vi "FL24 Dryer Tool Main.vi"() -> ()   [LabVIEW 2016]
uses:
  Q:/Common/LabVIEW GEA2 Toolkit/LabVIEW_GEA2_Toolkit.lvlibp/type defs/Data In.ctl
  Q:/Common/LabVIEW GEA2 Toolkit/LabVIEW_GEA2_Toolkit.lvlibp/type defs/Source_Destination.ctl
  Q:/Common/LabVIEW GEA2 Toolkit/LabVIEW_GEA2_Toolkit.lvlibp/type defs/Data Type.ctl
  Q:/Common/LabVIEW GEA2 Toolkit/LabVIEW_GEA2_Toolkit.lvlibp/type defs/ERD Read Data In.ctl
  Q:/MyWork/TL24 Tool/Laundry Tool 2.0 Support/type defs2/Select _Graph_Brass.ctl
  Q:/MyWork/TL24 Tool/Laundry Tool 1.0 Support/type defs/ERD_Graph_All.ctl
  Q:/MyWork/TL24 Tool/Laundry Tool 1.0 Support/type defs/ERD_Graph.ctl
  Q:/MyWork/TL24 Tool/Laundry Tool 1.0 Support/type defs/Version.ctl
  Q:/MyWork/TL24 Tool/Laundry Tool 2.0 Support/type defs2/ERD_Always_Show_Brass.ctl
  Q:/MyWork/TL24 Tool/Laundry Tool 1.0 Support/type defs/Fault_Buffer_Status.ctl
  Q:/MyWork/TL24 Tool/Laundry Tool 2.0 Support/type defs2/Diagnostics_Table.ctl
  Q:/MyWork/TL24 Tool/Laundry Tool 1.0 Support/type defs/Cycle_Diag_Buffer_Status.ctl
  Q:/MyWork/TL24 Tool/Laundry Tool 2.0 Support/type defs2/ERD_Data_Loop_Control_Brass.ctl
  Q:/MyWork/TL24 Tool/Laundry Tool 2.0 Support/type defs2/ERD_Loop_States_Brass.ctl
  Q:/MyWork/TL24 Tool/Laundry Tool 2.0 Support/type defs2/Error_Command_Brass.ctl
  Q:/MyWork/TL24 Tool/Laundry Tool 2.0 Support/type defs2/DAQ_States_Brass.ctl
  Q:/Common/GExplorer Support/typedefs/GExplorer_Data_Cluster.ctl
  Q:/MyWork/TL24 Tool/Laundry Tool 1.0 Support/type defs/Cont_Send_States.ctl
  Q:/MyWork/TL24 Tool/Laundry Tool 2.0 Support/type defs2/Cont_Send_States_Brass.ctl
  Q:/Common/LabVIEW GEA2 Toolkit/LabVIEW_GEA2_Toolkit.lvlibp/type defs/Data Out.ctl
  Q:/Common/LabVIEW GEA2 Toolkit/LabVIEW_GEA2_Toolkit.lvlibp/type defs/ERD Write Data In.ctl
  Q:/MyWork/TL24 Tool/Laundry Tool 2.0 Support/type defs2/DAQ_Control_Command_Brass.ctl
  Q:/MyWork/TL24 Tool/Laundry Tool 2.0 Support/type defs2/ERD_Loop_Control_Command_Brass.ctl
  Q:/MyWork/TL24 Tool/Laundry Tool 2.0 Support/type defs2/GEA2_Control_Command_Brass.ctl
  <vilib>/DAQmx/read.llb/DAQmx Read (Digital 1D Bool NChan 1Samp 1Line).vi
  <vilib>/DAQmx/read.llb/DAQmx Read (Digital 1D U8 1Chan NSamp).vi
  <vilib>/DAQmx/write.llb/DAQmx Write (Digital Bool 1Line 1Point).vi
  <vilib>/DAQmx/read.llb/DAQmx Read (Counter U32 1Chan 1Samp).vi
  <vilib>/DAQmx/write.llb/DAQmx Write (Analog 1D DBL NChan 1Samp).vi
  <vilib>/DAQmx/write.llb/DAQmx Write (Digital 1D Bool NChan 1Samp 1Line).vi
  Q:/Common/LabVIEW GEA2 Toolkit/LabVIEW_GEA2_Toolkit.lvlibp/advanced/GEA2 Message Received Event Handler.vi
  <vilib>/DAQmx/create/channels.llb/DAQmx Create Channel (DO-Digital Output).vi
  <vilib>/DAQmx/create/channels.llb/DAQmx Create Channel (DI-Digital Input).vi
  <vilib>/DAQmx/configure/timing.llb/DAQmx Timing (Sample Clock).vi
  <vilib>/DAQmx/create/channels.llb/DAQmx Create Channel (CO-Pulse Generation-Frequency).vi
  <vilib>/DAQmx/configure/timing.llb/DAQmx Timing (Implicit).vi
  <vilib>/DAQmx/create/channels.llb/DAQmx Create Channel (CI-Count Edges).vi
  <vilib>/DAQmx/create/channels.llb/DAQmx Create Channel (AO-Voltage-Basic).vi
  <vilib>/DAQmx/miscellaneous.llb/DAQmx Fill In Error Info.vi
  C:/Automation/DLLs/PC Dot Net/GeaCommunication.dll
  Automation/DLLs/PC Dot Net/GeaCommunication.dll
  Q:/Common/LabVIEW GEA2 Toolkit/LabVIEW_GEA2_Toolkit.lvlibp
  Q:/Automation/Product Specific/Clothes Care/2015 VA Washer/Projects/2015 VA Washer.lvlib
  <resource>/objmgr/daqmx.rc
panel:
  in  "Data ON":bool=TRUE
  out "ERD_Always Show":T1
  in  "Stop":bool
  out "Fault Status":bool
  out "Log Rate (ms)":u32
  in  "Tab Control":T2(tab)
  in  "Filter Data":bool=TRUE
  in  "Start Send":bool
  in  "Cmd":string
  in  "Filter Log":bool
  in  "Msg Rate (ms)":u32=1000 min=50 step=50
  out "CSV File Log Path":path=path "C:/Users/502129737/Desktop/1"
  in  "Clear":bool
  out "GEA2 Log":string
  in  "Board Index":u8 max=0 step=1
  out "Board ID":string="0"
  in  "GEA2 Send":T3={"Source"=228, "Destination"=53, "Command"=0, "Message"=""} {"Command" format="%02x"; "Destination" format="%02x"; "Source" format="%02x"}
  in  "Send Button":bool
  in  "GEA2 Log Length":i32=100000
  in  "Save Log":bool
  out "Version":T4
  in  "GEA Inputs":T5={"Source"=228, "Destination"=53} {"Destination" format="%.0x"; "Source" format="%.0x"}
  in  "Read ERD List":T6[](array[typedef])=[{"ERD Number"=0, "Data Type"=enum."string"}] {"ERD Number" format="%.0x"}
  out "Read ERD Data Out":cluster{"ERD Number":u16, "Data":string}[](array[cluster]) {"ERD Number" format="%.0x"}
  in  "Read ERD":bool
  in  "Write ERD":bool
  in  "Write ERD List":T8(array[cluster])=[{"ERD Number"=0, "Data Type"=enum."string", "Data"=""}] {"ERD Number" format="%.0x"}
  out "All Loads":u16[][](graph)=[[0, 100, 200, 300, 400]]
  in  "ERD Graphing ON":bool
  out "ERD Graph  Ind":T9
  in  "ERD Graph Cntrl":T10={"ERD 3"={"ERD #"=62250, "Data Type"=enum."uint16_t", "Scaler"=32}, "ERD 2"={"ERD #"=62250, "Data Type"=enum."uint16_t", "Scaler"=32}, "ERD 1"={"ERD #"=62250, "Data Type"=enum."uint16_t", "Scaler"=32}} {"ERD 1"."Scaler" min=1; "ERD 1"."ERD #" format="%.0x"; "ERD 2"."Scaler" min=1; "ERD 2"."ERD #" format="%.0x"; "ERD 3"."Scaler" min=1; "ERD 3"."ERD #" format="%.0x"}
  in  "Graphing ON":bool=TRUE
  in  "Select Graph":T12
  out "ERD 3":dbl(graph)
  out "ERD 2":dbl(graph)
  out "ERD 1":dbl(graph)
  in  "Save Fault Log":bool
  in  "Clear Fault Table Buffer":bool
  in  "Clear Fault Seq Buffer":bool
  in  "Fault ON":bool
  out "Fault Table Buffer":string[][](table)
  out "Fault Sequence Buffer":string
  out "Seq Buffer Status":T13
  out "Table Buffer Status":T13
  in  "Save Cycle History Log":bool
  in  "Clear Cycle Buffer":bool
  out "Cycle Buffer Status":T14
  in  "Get Cycle History":bool
  out "Diagnostics Table":T15
  in  "Test Mode":cluster{"Exit":bool, "Enter":bool}
  in  "Lid Lock":cluster{"Lock Lid":bool, "Unlock Lid":bool}
  in  "HE/LE ?":enum16{"HE", "LE"}(ring)
  in  "LL (M - A)":bool=TRUE
  in  "Lid Lock Feedback":bool
  in  "MS (M - A)":bool=TRUE
  out "DAQ Status":string
  out "Drain Pump":bool
  out "Mode Shift":bool
  out "Recirc Pump":bool
  out "Cold Valve":bool
  out "Hot Valve":bool
  out "Spray/Rinse Valve":bool
  out "Fabric SoftValve":bool
  in  "AC Power":bool=TRUE
  in  "Mode Shift FB":bool
  in  "Lid Status":bool=TRUE
  in  "Pressure":dbl(slide) min=0.0 max=5.0 step=0.5 scale=0.0..5.0 scale format="%#_3g"
  in  "Motor Current":dbl(slide)=2.5 min=0.0 max=5.0 step=0.5 scale=0.0..5.0 scale format="%#_3g"
  in  "Turn On DAQ":bool
  out "DAQ On?":bool
  in  "Basket RPM":dbl=1.0 min=1.0 max=800.0 step=5.0
  in  "Temperature":dbl(slide)=2.5 min=0.0 max=5.0 step=0.5 scale=0.0..5.0 scale format="%#_3g"
  out "Triac CW":bool
  out "Traic CCW":bool
  out "CCW":u32
  out "CW":u32
  in  "ERD Read List":T16(array[cluster])=[{"Boolean"=TRUE, "ERD Number"=1, "ERD Name"="Model Number", "Data Type"=enum."string"}, {"Boolean"=TRUE, "ERD Number"=2, "ERD Name"="Serial Number", "Data Type"=enum."string"}, {"Boolean"=TRUE, "ERD Number"=8192, "ERD Name"="Machine Status", "Data Type"=enum."uint8_t"}, {"Boolean"=TRUE, "ERD Number"=8202, "ERD Name"="Cycle Name", "Data Type"=enum."string"}, {"Boolean"=TRUE, "ERD Number"=142, "ERD Name"="Cycle Count", "Data Type"=enum."uint32_t"}, {"Boolean"=TRUE, "ERD Number"=8193, "ERD Name"="Sub-Cycle", "Data Type"=enum."string"}, {"Boolean"=TRUE, "ERD Number"=141, "ERD Name"="System Runtime", "Data Type"=enum."uint32_t"}, {"Boolean"=TRUE, "ERD Number"=8208, "ERD Name"="Delay Time", "Data Type"=enum."uint16_t"}, {"Boolean"=FALSE, "ERD Number"=256, "ERD Name"="Version", "Data Type"=enum."string"}, {"Boolean"=TRUE, "ERD Number"=70, "ERD Name"="Cycle Time", "Data Type"=enum."uint16_t"}, {"Boolean"=TRUE, "ERD Number"=8206, "ERD Name"="Operating Mode", "Data Type"=enum."string"}, {"Boolean"=TRUE, "ERD Number"=8210, "ERD Name"="Door Status", "Data Type"=enum."string"}, {"Boolean"=TRUE, "ERD Number"=8217, "ERD Name"="Temp Level", "Data Type"=enum."string"}, {"Boolean"=TRUE, "ERD Number"=8218, "ERD Name"="Dryness Level", "Data Type"=enum."string"}, {"Boolean"=TRUE, "ERD Number"=8219, "ERD Name"="Extended Tumble", "Data Type"=enum."string"}, {"Boolean"=TRUE, "ERD Number"=61445, "ERD Name"="Input Status", "Data Type"=enum."string"}, {"Boolean"=TRUE, "ERD Number"=61444, "ERD Name"="Dryer Type", "Data Type"=enum."string"}] {"ERD Number" format="%.0x"}
  out "Error Out":errorcluster
  in  "Error In":errorcluster
  # "Software Version"
  # "UI"
  # "MC"
  # "Must input a valid ERD# and Data Type\nDO NOT Leave Blank \nIf no scaler use value of 01"
  # "Contact:\n\nDerek Hibdon\nderek.hibdon@ge.com"
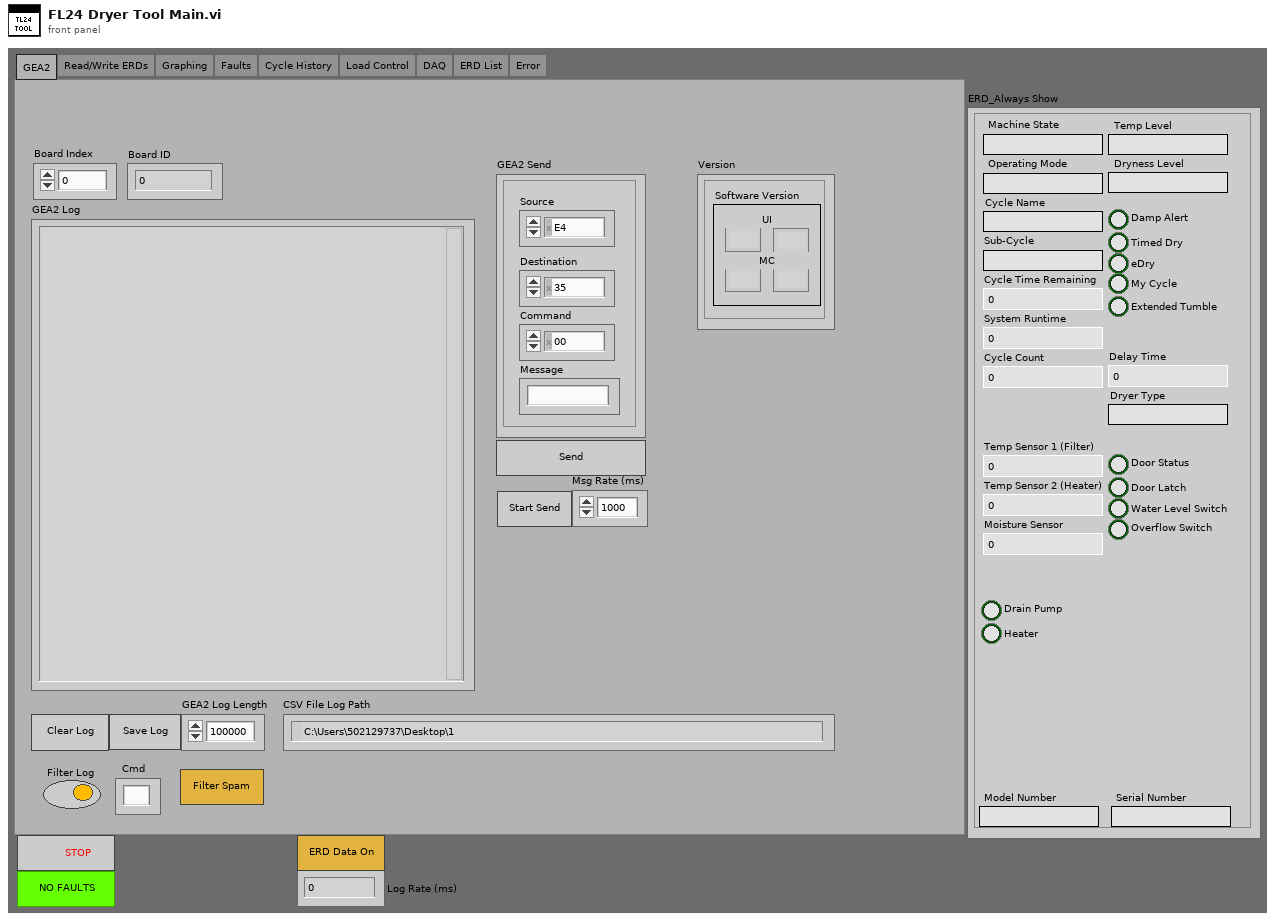
[diagram p1: front panel]
types:
  T1 = typedef "ERD_Always_Show_Brass.ctl" = cluster{"Machine State":string, "Cycle Count":u32, "Dryness Level":string, "Temp Level":string, "Delay Time":u16, "Sub-Cycle":string, "Cycle Name":string, "Model Number":string, "Serial Number":string, "System Runtime":u32, "Cycle Time Remaining":u16, "Operating Mode":string, "Temp Sensor 1 (Filter)":u16, "Drain Pump":bool, "Water Level Switch":bool, "Overflow Switch":bool, "Door Status":bool, "Door Latch":bool, "Heater":bool, "Temp Sensor 2 (Heater)":u16, "Moisture Sensor":u16, "Dryer Type":string, "eDry":bool, "Damp Alert":bool, "Timed Dry":bool, "My Cycle":bool, "Extended Tumble":bool}
  T2 = enum32{"GEA2", "Read/Write ERDs", "Graphing", "Faults", "Cycle History", "Load Control", "DAQ", "ERD List", "Error"}
  T3 = typedef "LabVIEW_GEA2_Toolkit.lvlibp/Data In.ctl" = cluster{"Source":u8, "Destination":u8, "Command":u8, "Message":string}
  T4 = typedef "Version.ctl" = cluster{"Critical Major":string, "Critical Minor":string, "Non-Critical Minor":string, "Non-Critical Major":string}
  T5 = typedef "LabVIEW_GEA2_Toolkit.lvlibp/Source_Destination.ctl" = cluster{"Source":u8, "Destination":u8}
  T6 = typedef "LabVIEW_GEA2_Toolkit.lvlibp/ERD Read Data In.ctl" = cluster{"ERD Number":u16, "Data Type":T7}
  T7 = typedef "LabVIEW_GEA2_Toolkit.lvlibp/Data Type.ctl" = enum16{"string", "boolean", "uint8_t", "uint16_t", "uint32_t", "uint64_t", "int8_t", "int16_t", "int32_t", "int64_t"}
  T8 = cluster{"ERD Number":u16, "Data Type":T7, "Data":string}[]
  T9 = cluster{"ERD Value 1":dbl, "ERD Value 2":dbl, "ERD Value 3":dbl}
  T10 = typedef "ERD_Graph_All.ctl" = cluster{"ERD 3":T11, "ERD 2":T11, "ERD 1":T11}
  T11 = typedef "ERD_Graph.ctl" = cluster{"ERD #":u16, "Data Type":T7, "Scaler":u32}
  T12 = typedef "Select _Graph_Brass.ctl" = enum16{"All Loads", "ERD 1", "ERD 2", "ERD 3", "Temperature (F)", "Basket Speed (RPM)", "Tub Volume (Gal)", "Pressure (in H2O)", "Current RMS (Amps)"}
  T13 = typedef "Fault_Buffer_Status.ctl" = cluster{"Current Index":u16, "Count":u16, "Overwrite Count":u16}
  T14 = typedef "Cycle_Diag_Buffer_Status.ctl" = cluster{"Current Index":u16, "Count":u16, "Overwrite Count":u16}
  T15 = typedef "Diagnostics_Table.ctl" = string[][]
  T16 = cluster{"Boolean":bool, "ERD Number":u16, "ERD Name":string, "Data Type":enum16{"string", "boolean", "uint8_t", "uint16_t", "uint32_t", "uint64_t"}}[]
  T17 = typedef "Cont_Send_States_Brass.ctl" = enum16{"Run", "Shutdown"}
  T18 = typedef "Cont_Send_States.ctl" = enum16{"Run", "Shutdown"}
  T19 = typedef "GExplorer_Data_Cluster.ctl" = cluster{"Data":variant, "State":enum16{"Add to Log", "Clear", "Shutdown"}}
  T20 = typedef "DAQ_States_Brass.ctl" = enum16{"Wait for Init", "Rename Devices", "Verify Hardware", "Initialize", "Run", "Shutdown", "Exit"}
  T21 = typedef "ERD_Data_Loop_Control_Brass.ctl" = cluster{"Data":variant, "State":T22}
  T22 = typedef "ERD_Loop_States_Brass.ctl" = enum16{"Init", "Build ERD Read List", "Read ERDs", "Update UI", "Update Graphs", "Read Faults", "Log Data", "Pause", "Shutdown"}
  T23 = typedef "Error_Command_Brass.ctl" = enum16{"Initialize", "Handle Errors", "Report Errors"}
  T24 = typedef "LabVIEW_GEA2_Toolkit.lvlibp/ERD Write Data In.ctl" = cluster{"ERD Number":u16, "Data Type":T7, "Data":string}
  T25 = typedef "GEA2_Control_Command_Brass.ctl" = enum16{"Initialize", "Shutdown"}
  T26 = typedef "ERD_Loop_Control_Command_Brass.ctl" = enum16{"Initialize", "Shutdown"}
  T27 = typedef "DAQ_Control_Command_Brass.ctl" = enum16{"Initialize", "Shutdown", "Exit"}
  T28 = enum8{"Enabled", "Disabled", "Disabled and Grayed Out"}
  T29 = typedef "LabVIEW_GEA2_Toolkit.lvlibp/Data Out.ctl" = cluster{"Source":u8, "Destination":u8, "Command":u8, "Length":u8, "CRC":u16, "Message":string}
  T30 = typedef "LabVIEW_GEA2_Toolkit.lvlibp/ERD Read Data Out.ctl" = cluster{"ERD Number":u16, "Data":string}
  T31 = typedef "All_Bundled_Data_Brass.ctl" = cluster{"Version":T4, "ERD_Always Show":T1, "Personality Set":u8, "CSV File String Arrays":T32, "Fault Table Array ":T33}
  T32 = typedef "CSV_File_String_Arrays.ctl" = cluster{"ERD Number Array":string[], "ERD Name Array":string[], "ERD Converted String Data":string[]}
  T33 = typedef "Fault Table Array.ctl" = T34[]
  T34 = typedef "Fault_Table_Info.ctl" = cluster{"Cycle Count":u32, " Runtime (min) ":u32, "Fault Status":string, "Fault ID":string, "Fault Count":u16}
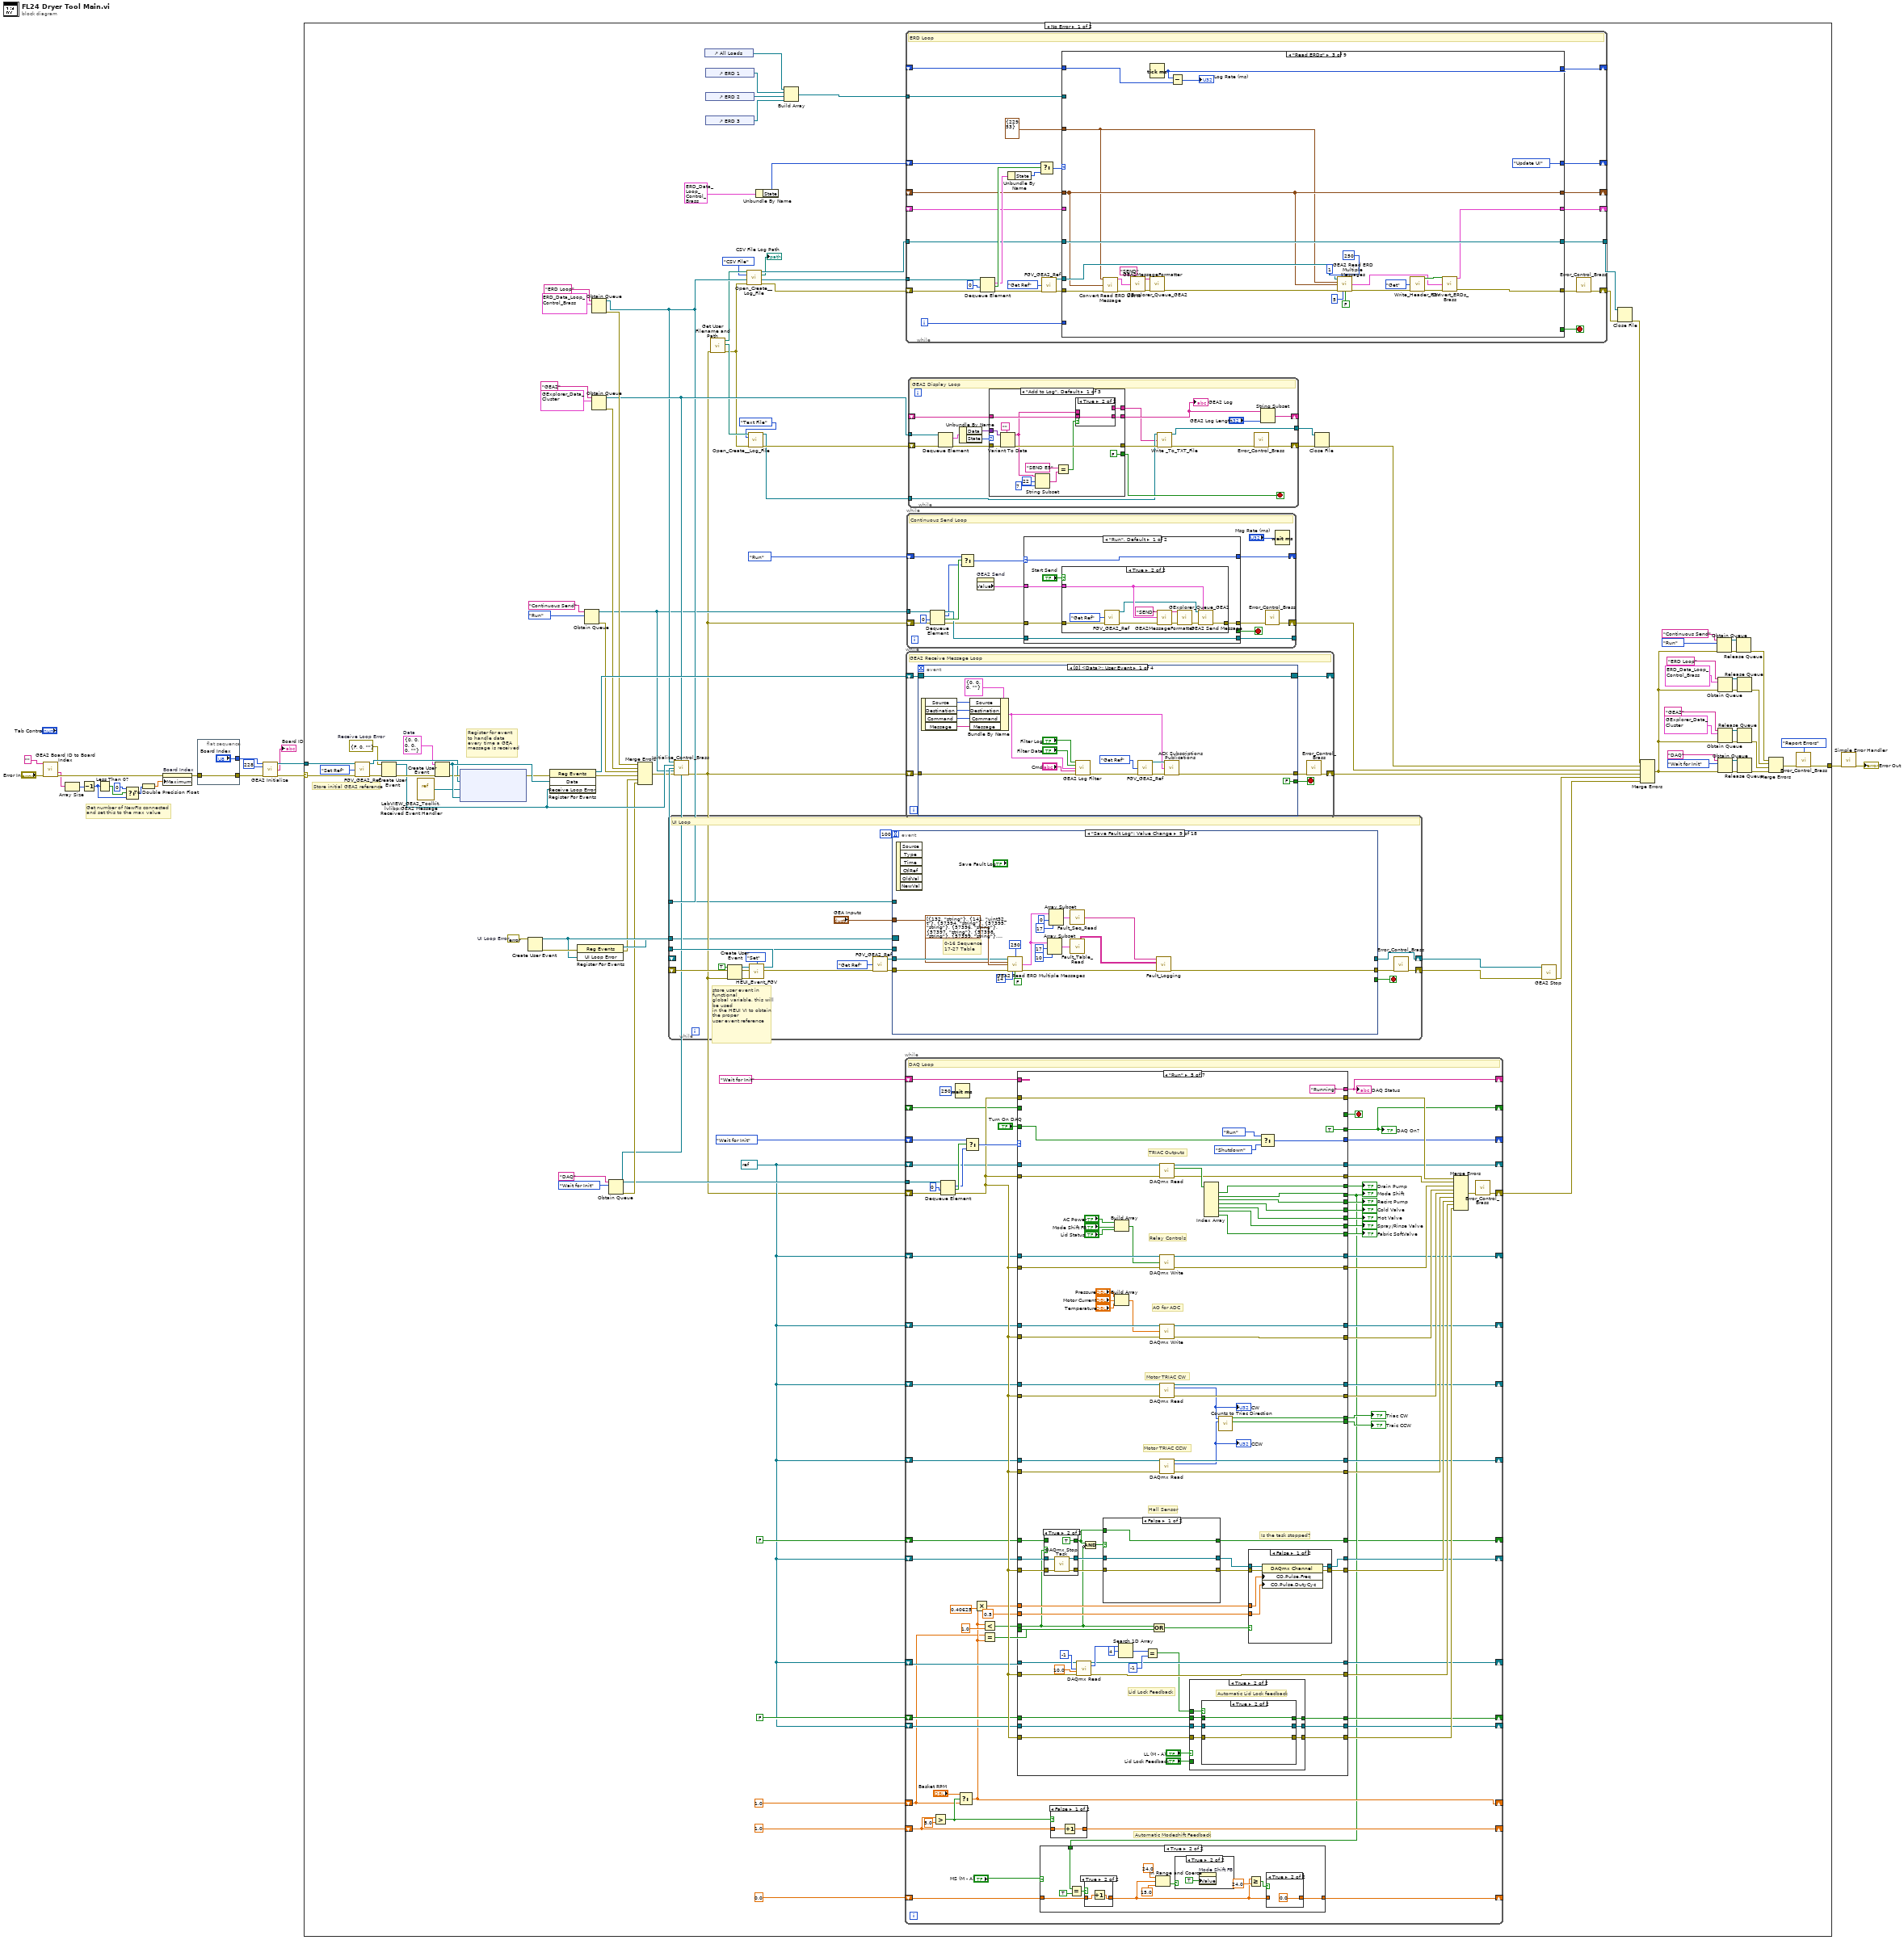
[diagram p0: block diagram]
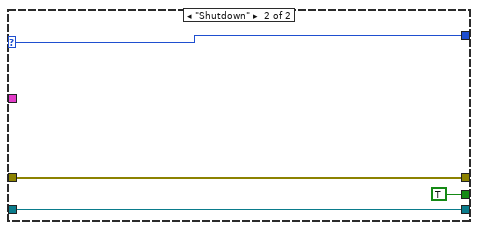
[diagram p3: hidden frame]
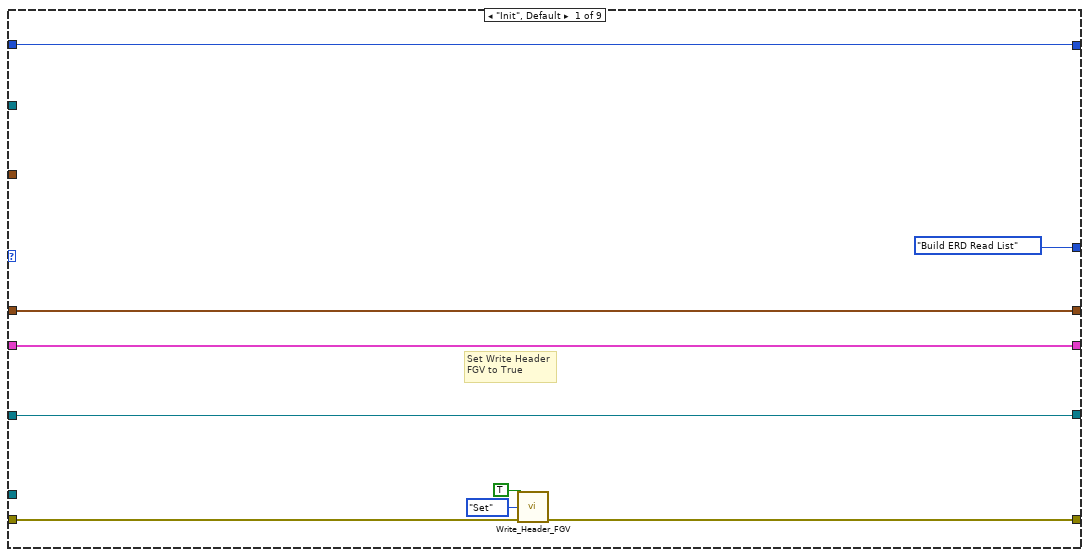
[diagram p4: hidden frame]
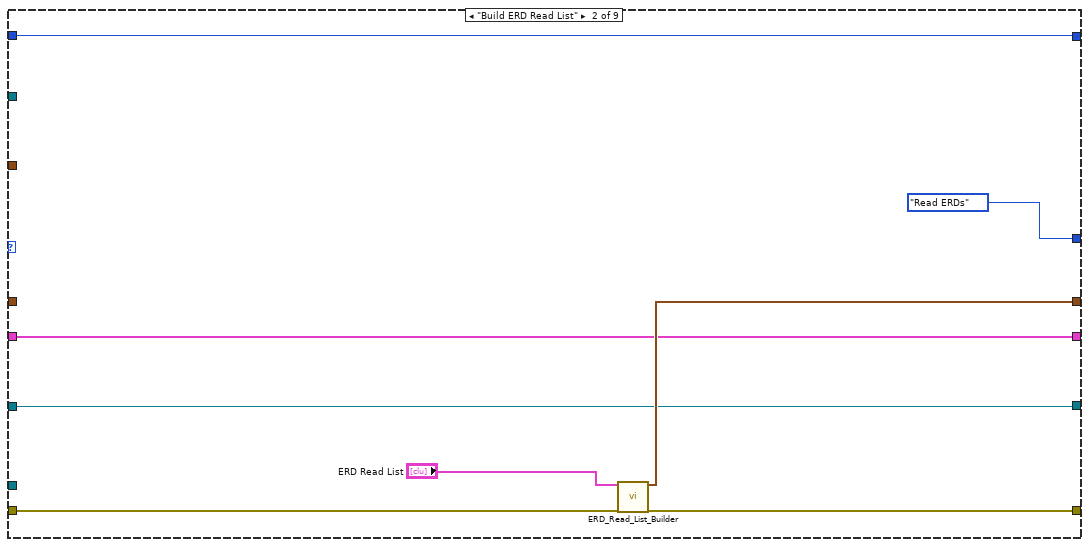
[diagram p5: hidden frame]
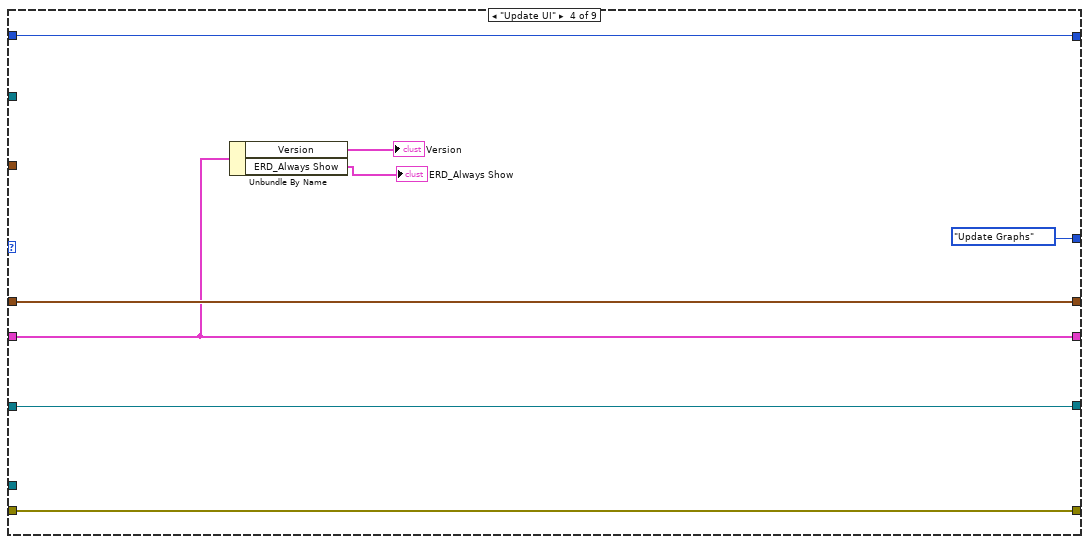
[diagram p6: hidden frame]
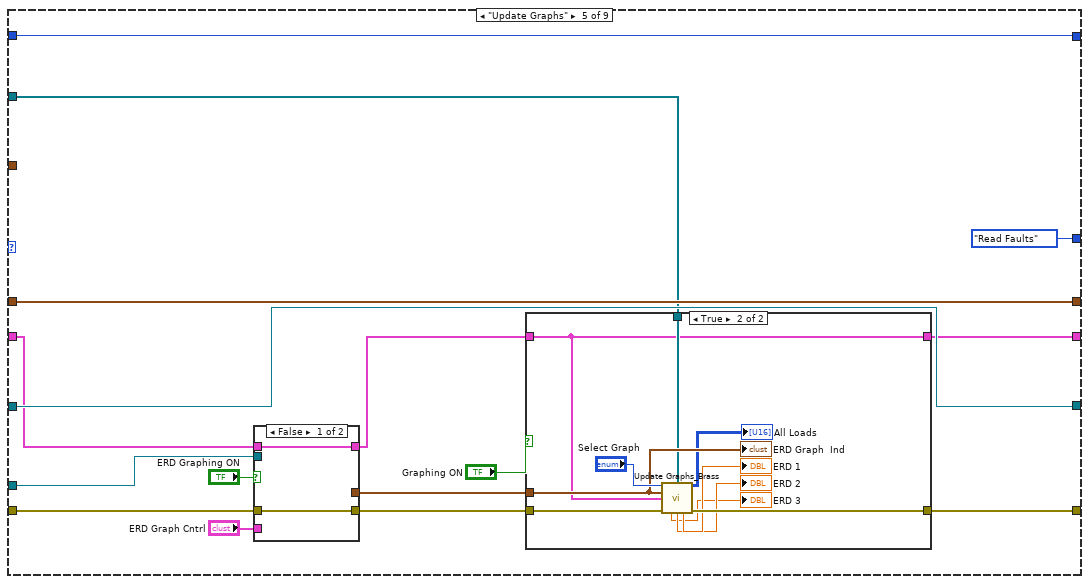
[diagram p7: hidden frame]
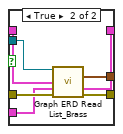
[diagram p9: hidden frame]
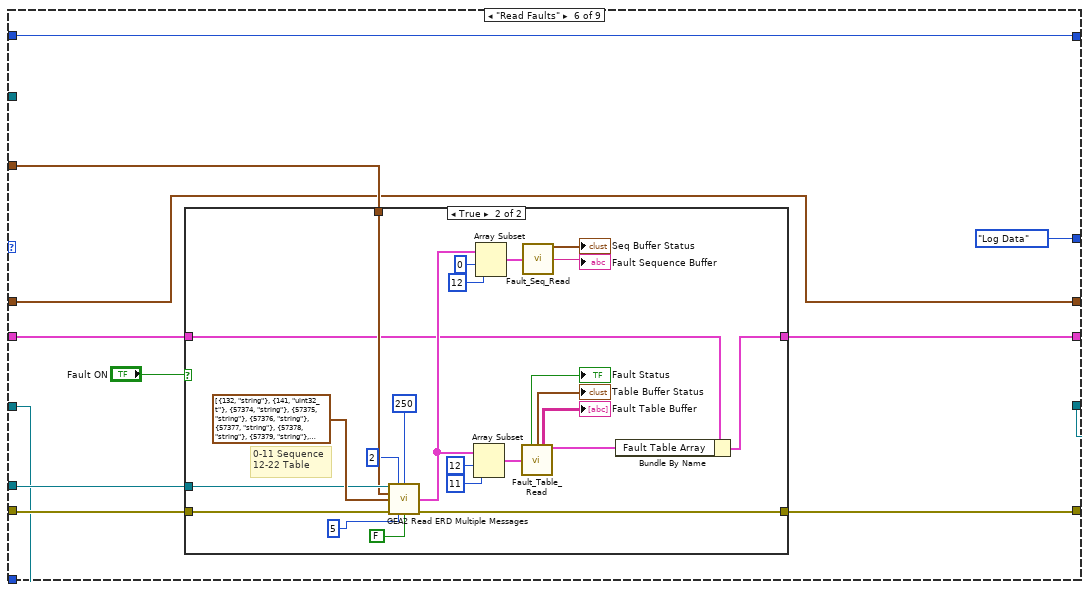
[diagram p10: hidden frame]
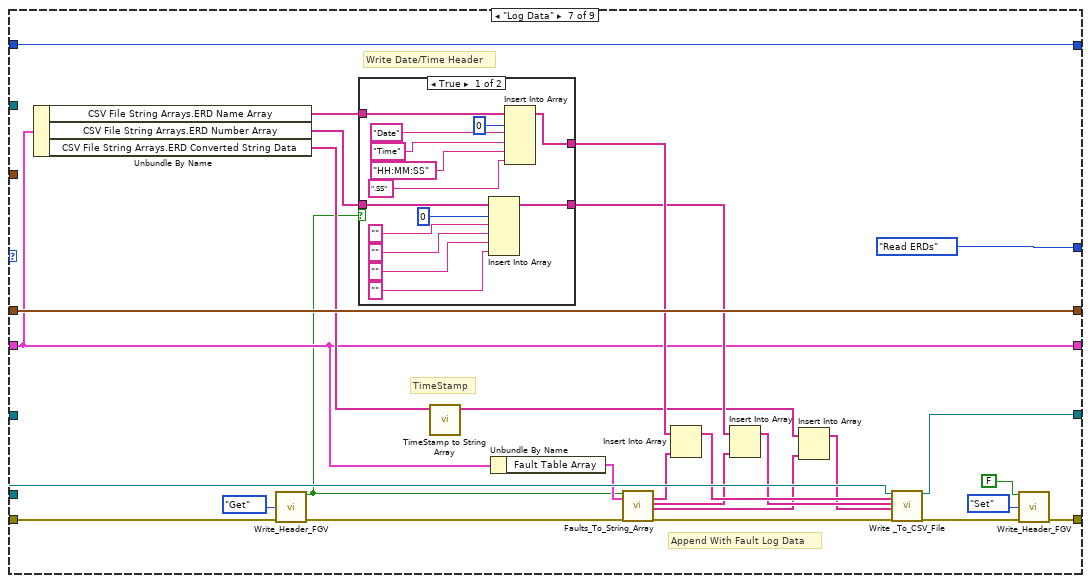
[diagram p12: hidden frame]
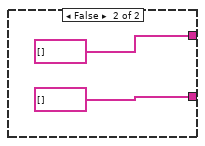
[diagram p13: hidden frame]
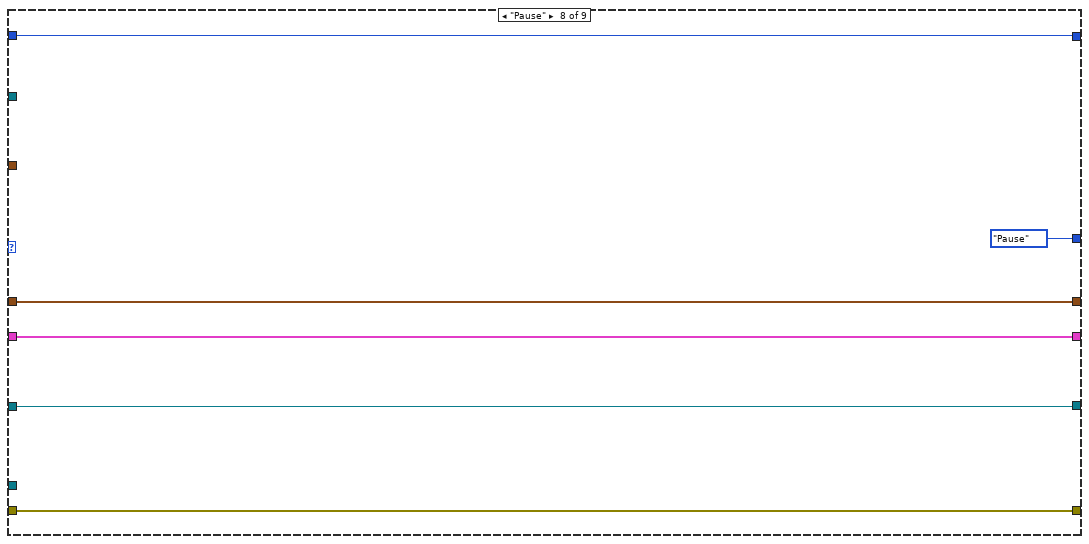
[diagram p14: hidden frame]
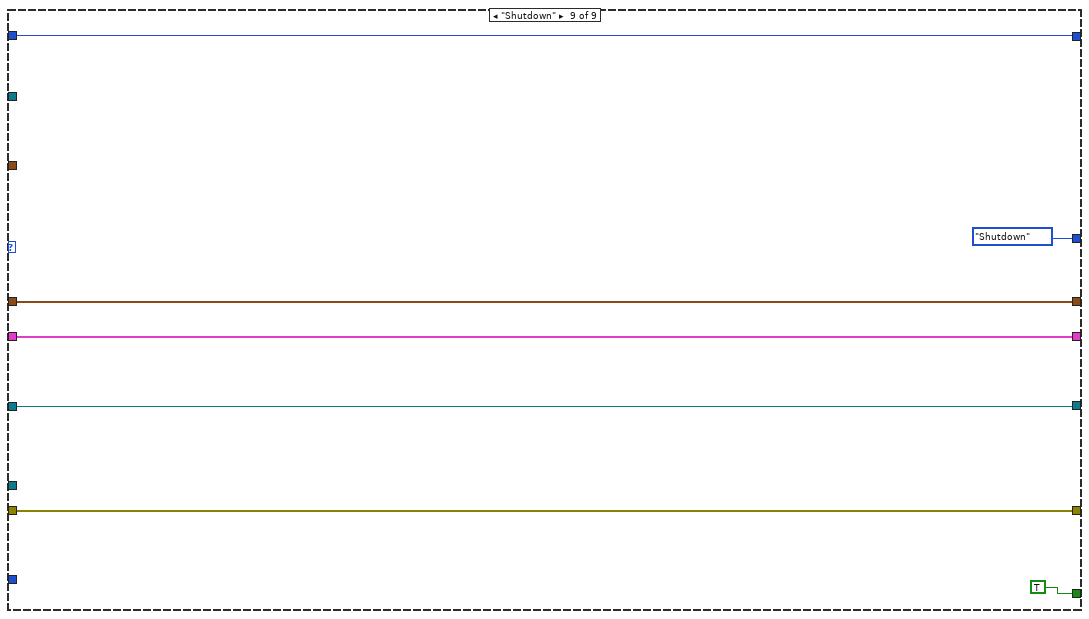
[diagram p15: hidden frame]
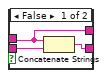
[diagram p16: hidden frame]
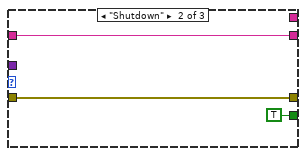
[diagram p17: hidden frame]
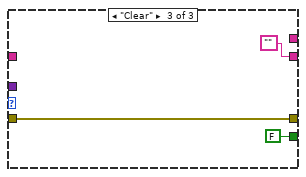
[diagram p18: hidden frame]
diagram:
  # "Get number of NewFIs connected\nand set this to the max value"
  n1 = call "GEA2 Board ID to Board Index.vi"("Board ID"="", "Error In"="Error In") -> ("Boards Found"=w4:string[], "Error Out"=w13:errorcluster)  [unwired: 9 in, 3 out]
  n2 = Array Size(array=w4) -> (size(s)=w9:i32)
  n3 = Decrement(x=w9) -> (x-1=w7:i32)
  n4 = Less Than 0?(x=w7) -> (x < 0?=w8:bool)
  n5 = Select(t=0, s=w8, f=w7) -> (s? t:f=w5:i32)
  n6 = To Double Precision Float(number=w5) -> (double precision float=w3:dbl)
  n7 = property on="Board Index" class="DigNum (strict)"(error in=w13, "Maximum"=w3) -> (error out=w11:errorcluster)  [unwired: 1 in, 1 out]
  n8 = flat-sequence {
    tunnel: ["Board Index"] -> w16
    tunnel: w11 -> [w20]
    tunnel: [w20] -> w10
    frame #0 {
    }
  }
  n9 = call "GEA2 Initialize.vi"("Board Index"=w16, "Source Address"=u8 228, "error in"=w10) -> ("GEA2 Reference Out"=w18:refnum<k24>, "Board ID"=→"Board ID":string, "error out"=w17:errorcluster)  [unwired: 10 in]
  n10 = case shown="No Error" w17 {
    selector: w17 -> [w81 w1348]
    tunnel: w18 -> [w79 _]
    tunnel: [w83 w1348] -> w2
    frame No Error {
      w35 = errorcluster {"status"=FALSE, "code"=0, "source"=""}  # Receive Loop Error
      w36 = T29 {"Source"=0, "Destination"=0, "Command"=0, "Length"=0, "CRC"=0, "Message"=""}  # Data
      w51 = refnum<k21> refnum ("task out")
      w117 = errorcluster {"status"=FALSE, "code"=0, "source"=""}  # UI Loop Error
      # "store user event in functional\nglobal variable, this will be used\nin the HEUI VI to obtain the proper\nuser event reference"
      # "Store initial GEA2 reference"
      # "Register for event\nto handle data\nevery time a GEA\nmessage is received"
      n11 = call "FGV_GEA2_Ref.vi"("GEA2 Reference In"=w79, "Action"=enum16{"Set Ref", "Get Ref"}."Set Ref", "Error In"=w81) -> ("GEA2 Reference Out"=w78:refnum<k24>, "Error Out"=w80:errorcluster)  [unwired: 11 in]
      n12 = Create User Event(user event datatype=w35, error in=w80) -> (user event=w118:refnum<user-event>, error out=w120:errorcluster)
      n13 = vi-ref "LabVIEW_GEA2_Toolkit.lvlibp:GEA2 Message Received Event Handler.vi"() -> (w119:refnum<vi>)
      n14 = Create User Event(user event datatype=w36, error in=w120) -> (user event=w123:refnum<user-event>, error out=w122:errorcluster)
      n15 = node(w122, w78, w119, w123) -> (w121:errorcluster)  [unwired: 1 in, 1 out]
      n16 = Create User Event(user event datatype=w117) -> (user event=w106:refnum<user-event>, error out=w116:errorcluster)  [unwired: 1 in]
      n17 = register-events(error in=w121, w123, w118) -> (reference out=w115:refnum<event-registration>, error out=w88:errorcluster)  [unwired: 1 in]
      n18 = register-events(error in=w116, w106) -> (reference out=w97:refnum<event-registration>, error out=w87:errorcluster)  [unwired: 1 in]
      n19 = Obtain Queue(name (unnamed)="Continuous Send", element data type=Cont_Send_States_Brass."Run" ("State")) -> (queue out=w37:refnum<queue>, error out=w42:errorcluster)  [unwired: 3 in, 1 out]
      n20 = Obtain Queue(name (unnamed)="ERD Loop", element data type=T21 {"Data"=variant, "State"=enum."Read ERDs"} ("Data")) -> (queue out=w66:refnum<queue>, error out=w84:errorcluster)  [unwired: 3 in, 1 out]
      n21 = Obtain Queue(name (unnamed)="GEA2", element data type=T19 {"Data"=variant, "State"=enum."Add to Log"} ("Data")) -> (queue out=w67:refnum<queue>, error out=w89:errorcluster)  [unwired: 3 in, 1 out]
      n22 = Obtain Queue(name (unnamed)="DAQ", element data type=DAQ_States_Brass."Wait for Init" ("States")) -> (queue out=w59:refnum<queue>, error out=w86:errorcluster)  [unwired: 3 in, 1 out]
      n23 = Merge Errors(w84, w89, w42, w88, w87, w86) -> (w85:errorcluster)
      n24 = call "Initialize_Control_Brass.vi"("ERD Loop"=w66, "GEA2"=w67, "Receive Loop"=w118, "UI Loop Error"=w106, "Cont Send"=w37, "Error In"=w85, "DAQ"=w59) -> ("Error Out"=w32:errorcluster)  [unwired: 8 in]
      n25 = control-ref of="All Loads"() -> (w22:refnum<vi>)
      n26 = control-ref of="ERD 1"() -> (w63:refnum<vi>)
      n27 = control-ref of="ERD 2"() -> (w61:refnum<vi>)
      n28 = control-ref of="ERD 3"() -> (w62:refnum<vi>)
      n29 = call "Get User Filename and Path.vi"("error in (no error)"=w32) -> ("error out"=w24:errorcluster, "TXT File Path"=w30:path, "CSV File Path"=w33:path)  [unwired: 8 in]
      n30 = Create User Event(user event datatype=TRUE ("Bool"), error in=w32) -> (user event=w73:refnum<user-event>, error out=w74:errorcluster)
      n31 = call "Open_Create__Log_File.vi"("File Path Control"=w33, "Enum"=enum16{"CSV File", "Text File"}."CSV File", "Error In"=w24) -> ("refnum out"=w64:refnum<file>, "File Path"=→"CSV File Log Path":path, "Error Out"=w76:errorcluster)  [unwired: 10 in]
      n32 = call "Open_Create__Log_File.vi"("File Path Control"=w30, "Enum"=enum16{"CSV File", "Text File"}."Text File", "Error In"=w24) -> ("refnum out"=w29:refnum<file>, "Error Out"=w31:errorcluster)  [unwired: 10 in, 1 out]
      n33 = call "HEUI_Event_FGV.vi"("Event In"=w73, "Action"=enum16{"Get", "Set"}."Set", "Error In"=w74) -> ("Event Out"=w70:refnum<user-event>, "Error Out"=w71:errorcluster)  [unwired: 11 in]
      n34 = while "UI Loop" {
        shift-right: [w1012] -> w125
        shift-left: w71 -> [w1006]
        shift-right: [w1014] -> w124
        shift-left: _ -> [_]
        tunnel: w97 -> [w1013]
        tunnel: w70 -> [w1003]
        tunnel: w66 -> [w1002]
        stop <- w1011 stop-if-true
        # "UI Loop"
        n35 = call "FGV_GEA2_Ref.vi"("Action"=enum16{"Set Ref", "Get Ref"}."Get Ref", "Error In"=w1006) -> ("GEA2 Reference Out"=w1005:refnum<k24>, "Error Out"=w1007:errorcluster)  [unwired: 12 in]
        n36 = event shown="[8] \"Save Fault Log\": Value Change" {
          selector: w1013 -> [_ _ _ _ _ _ _ _ _ _ _ _ _ _ _ _ _ _]
          dyn-events: _ -> [_ _ _ _ _ _ _ _ _ _ _ _ _ _ _ _ _ _]
          timeout: 100 -> [_ _ _ _ _ _ _ _ _ _ _ _ _ _ _ _ _ _]
          tunnel: [w1020 w1030 w1031 w1037 w1051 w1061 w1074 w1081 w1084 w1103 _ _ w1206 w1225 w1239 w1257 w1277 w1288] -> w1010
          tunnel: w1007 -> [w1017 w1027 w1031 w1033 w1048 w1065 w1072 w1079 w1088 w1106 w1121 w1164 w1209 w1231 w1247 w1263 w1278 w1295]
          tunnel: [_ _ _ _ _ _ _ _ _ _ _ _ _ _ _ _ _ TRUE] -> w1011
          tunnel: w1005 -> [w1015 w1029 w1032 w1035 w1049 _ _ _ w1090 w1105 w1120 w1163 w1208 w1230 w1241 w1262 _ w1298]
          tunnel: [w1022 w1029 w1032 w1038 w1050 _ _ _ _ w1104 _ _ w1207 _ _ _ _ w1298] -> w1014
          tunnel: "GEA Inputs" -> [_ _ _ w1036 w1046 _ _ _ w1089 w1107 w1119 w1162 w1210 w1228 w1240 w1264 _ _]
          tunnel: w1003 -> [_ _ _ _ _ _ _ _ _ _ _ _ _ _ _ _ _ _]
          tunnel: w1002 -> [_ _ _ _ _ _ w1070 w1077 _ _ _ _ _ _ _ _ w1275 _]
          event "Send Button": Value Change {
            n37 = event-data() -> ()  [unwired: 1 in, 1 out]
            n38 = call "GEA2MessageFormatter.vi"("Prefix(Send/Recv)"="SEND", "GEA2 Data In"="GEA2 Send", "Error In"=w1017) -> ("Output String"=w1019:string, "Error Out"=w1018:errorcluster)  [unwired: 11 in]
            n39 = call "GExplorer_Queue_GEA2.vi"("Output String"=w1019, "error in (no error)"=w1018) -> ("error out"=w1021:errorcluster)  [unwired: 13 in]
            n40 = call "GEA2 Send Message.vi"("GEA2 Reference In"=w1015, "Input Data"="GEA2 Send", "Error In"=w1021) -> ("GEA2 Reference Out"=w1022:refnum<k24>, "Error Out"=w1020:errorcluster)  [unwired: 11 in]
          }
          event "Clear": Value Change {
            w1024 = T19 {"Data"=variant, "State"=enum."Clear"} ("element")
            n41 = event-data() -> ()  [unwired: 1 in, 6 out]
            n42 = Obtain Queue(name (unnamed)="GEA2", element data type=w1024, error in (no error)=w1027) -> (queue out=w1025:refnum<queue>, error out=w1028:errorcluster)  [unwired: 2 in, 1 out]
            n43 = Enqueue Element(queue=w1025, element=w1024, error in (no error)=w1028) -> (error out=w1030:errorcluster)  [unwired: 1 in, 2 out]
          }
          event Timeout {
            # "Must have timeout case to give GEA2 FGV a chance to update\nthe GEA2 reference. Otherwise, when we receive an event it may\nbe using a reference that is no longer valid."
            n44 = event-data() -> ()  [unwired: 1 in, 3 out]
          }
          event "Write ERD": Value Change {
            n45 = event-data() -> ()  [unwired: 1 in, 1 out]
            n46 = call "Convert Write ERD List to Message.vi"("GEA Inputs"=w1036, "Write ERD List"="Write ERD List", "Error In"=w1033) -> ("GEA Message"=w1042:T3, "Error Out"=w1043:errorcluster)  [unwired: 11 in]
            n47 = call "GEA2MessageFormatter.vi"("Prefix(Send/Recv)"="SEND", "GEA2 Data In"=w1042, "Error In"=w1043) -> ("Output String"=w1044:string, "Error Out"=w1045:errorcluster)  [unwired: 11 in]
            n48 = call "GExplorer_Queue_GEA2.vi"("Output String"=w1044, "error in (no error)"=w1045) -> ("error out"=w1040:errorcluster)  [unwired: 13 in]
            n49 = call "GEA2 Write ERD.vi"("GEA2 Reference In"=w1035, "GEA Inputs"=w1036, "Write ERD List"="Write ERD List", "Error In"=w1040, "Verify ERD Response?"=FALSE) -> ("GEA2 Reference Out"=w1038:refnum<k24>, "Error Out"=w1037:errorcluster)  [unwired: 8 in, 1 out]
          }
          event "Read ERD": Value Change {
            n50 = event-data() -> ()  [unwired: 1 in, 6 out]
            n51 = call "Convert Read ERD List to Message.vi"("GEA Inputs"=w1046, "Read ERD List"="Read ERD List", "Error In"=w1048) -> ("GEA Message"=w1056:T3, "Error Out"=w1047:errorcluster)  [unwired: 11 in]
            n52 = call "GEA2MessageFormatter.vi"("Prefix(Send/Recv)"="SEND", "GEA2 Data In"=w1056, "Error In"=w1047) -> ("Output String"=w1054:string, "Error Out"=w1053:errorcluster)  [unwired: 11 in]
            n53 = call "GExplorer_Queue_GEA2.vi"("Output String"=w1054, "error in (no error)"=w1053) -> ("error out"=w1057:errorcluster)  [unwired: 13 in]
            n54 = call "GEA2 Read ERD.vi"("GEA2 Reference In"=w1049, "GEA Inputs"=w1046, "Read ERD List"="Read ERD List", "Error In"=w1057, "Verify ERD Response?"=FALSE) -> ("GEA2 Reference Out"=w1050:refnum<k24>, "ERD Data Out"=→"Read ERD Data Out":T30[], "Error Out"=w1051:errorcluster)  [unwired: 7 in, 1 out]
          }
          event "Save Log": Value Change {
            n55 = event-data() -> ()  [unwired: 1 in, 6 out]
            n56 = property on="GEA2 Log" class="Str"(error in=w1065) -> (error out=w1067:errorcluster, "Value"=w1066:string)  [unwired: 1 in, 1 out]
            n57 = Write to Text File(prompt (Choose or enter file path)="Choose filename and path to save txt file to ", text=w1066, error in=w1067) -> (refnum out=w1064:refnum<file>, error out=w1063:errorcluster)  [unwired: 1 in, 1 out]
            n58 = Close File(refnum=w1064, error in=w1063) -> (error out=w1062:errorcluster)  [unwired: 1 out]
            n59 = call <vilib>:"Clear Errors.vi"("error in (no error)"=w1062, "specific error code to clear (0: all)"=43) -> ("error out"=w1061:errorcluster)  [unwired: 4 in, 1 out]
          }
          event "ERD Read List": Value Change {
            n60 = event-data() -> ()  [unwired: 1 in, 6 out]
            n61 = Enqueue Element(queue=w1070, element=T21 {"Data"=variant, "State"=enum."Build ERD Read List"}, error in (no error)=w1072) -> (error out=w1071:errorcluster)  [unwired: 1 in, 2 out]
            n62 = call "Write_Header_FGV.vi"("Write Header ? In"=TRUE, "Action"=enum16{"Get", "Set"}."Set", "Error In"=w1071) -> ("Error Out"=w1074:errorcluster)  [unwired: 11 in, 1 out]
          }
          event "Fault ON", "ERD Graphing ON": Value Change {
            n63 = event-data() -> ()  [unwired: 1 in, 6 out]
            n64 = Enqueue Element(queue=w1077, element=T21 {"Data"=variant, "State"=enum."Build ERD Read List"}, error in (no error)=w1079) -> (error out=w1078:errorcluster)  [unwired: 1 in, 2 out]
            n65 = call "Write_Header_FGV.vi"("Write Header ? In"=TRUE, "Action"=enum16{"Get", "Set"}."Set", "Error In"=w1078) -> ("Error Out"=w1081:errorcluster)  [unwired: 11 in, 1 out]
          }
          event "Save Fault Log": Value Change {
            # "0-16 Sequence\n17-27 Table"
            n66 = event-data() -> ()  [unwired: 1 in, 6 out]
            n67 = call "GEA2 Read ERD Multiple Messages.vi"("GEA2 Reference In"=w1090, "Read Timeout (ms)"=u32 250, "GEA Inputs"=w1089, "Read ERD List"=T6[] [{"ERD Number"=132, "Data Type"=enum."string"}, {"ERD Number"=141, "Data Type"=enum."uint32_t"}, {"ERD Number"=57394, "Data Type"=enum."string"}, {"ERD Number"=57395, "Data Type"=enum."string"}, {"ERD Number"=57396, "Data Type"=enum."string"}, {"ERD Number"=57397, "Data Type"=enum."string"}, {"ERD Number"=57398, "Data Type"=enum."string"}, {"ERD Number"=57399, "Data Type"=enum."string"}, {"ERD Number"=57400, "Data Type"=enum."string"}, {"ERD Number"=57401, "Data Type"=enum."string"}, {"ERD Number"=57402, "Data Type"=enum."string"}, {"ERD Number"=57403, "Data Type"=enum."string"}, {"ERD Number"=57404, "Data Type"=enum."string"}, {"ERD Number"=57405, "Data Type"=enum."string"}, {"ERD Number"=57406, "Data Type"=enum."string"}, {"ERD Number"=57407, "Data Type"=enum."string"}, {"ERD Number"=57408, "Data Type"=enum."string"}, {"ERD Number"=129, "Data Type"=enum."string"}, {"ERD Number"=57444, "Data Type"=enum."string"}, {"ERD Number"=57445, "Data Type"=enum."string"}, {"ERD Number"=57446, "Data Type"=enum."string"}, {"ERD Number"=57447, "Data Type"=enum."string"}, {"ERD Number"=57448, "Data Type"=enum."string"}, {"ERD Number"=57449, "Data Type"=enum."string"}, {"ERD Number"=57450, "Data Type"=enum."string"}, {"ERD Number"=57451, "Data Type"=enum."string"}, {"ERD Number"=57452, "Data Type"=enum."string"}, {"ERD Number"=57453, "Data Type"=enum."string"}], "Error In"=w1088, "#ERDs per message"=14 ("#ERDs per message 2"), "Verify ERD Response?"=FALSE) -> ("ERD Data Out"=w1093:T30[], "Error Out"=w1085:errorcluster)  [unwired: 5 in, 2 out]
            n68 = Array Subset(array=w1093, index=17, length=10) -> (w1094:T30[])
            n69 = Array Subset(array=w1093, index=0, length=17) -> (w1092:T30[])
            n70 = call "Fault_Seq_Read.vi"("Seq ERD In"=w1092) -> ("String"=w1087:string)  [unwired: 13 in, 1 out]
            n71 = call "Fault_Table_Read.vi"("ERD Data Out"=w1094) -> ("Fault Table String Out"=w1086:string[][])  [unwired: 11 in, 3 out]
            n72 = call "Fault_Logging.vi"("String"=w1087, "Fault Table String Out"=w1086, "error in (no error)"=w1085) -> ("error out"=w1084:errorcluster)  [unwired: 12 in]
          }
          event "Clear Fault Seq Buffer": Value Change {
            n73 = event-data() -> ()  [unwired: 1 in, 6 out]
            n74 = Bundle By Name(cluster=T24 {"ERD Number"=133, "Data Type"=enum."string", "Data"=""} ("ERD Read Data In"), "Data"="FF") -> (w1116:T24)
            n75 = Build Array(w1116) -> (w1110:T24[])
            n76 = call "Convert Write ERD List to Message.vi"("GEA Inputs"=w1107, "Write ERD List"=w1110, "Error In"=w1106) -> ("GEA Message"=w1112:T3, "Error Out"=w1113:errorcluster)  [unwired: 11 in]
            n77 = call "GEA2MessageFormatter.vi"("Prefix(Send/Recv)"="SEND", "GEA2 Data In"=w1112, "Error In"=w1113) -> ("Output String"=w1114:string, "Error Out"=w1115:errorcluster)  [unwired: 11 in]
            n78 = call "GExplorer_Queue_GEA2.vi"("Output String"=w1114, "error in (no error)"=w1115) -> ("error out"=w1111:errorcluster)  [unwired: 13 in]
            n79 = call "GEA2 Write ERD.vi"("GEA2 Reference In"=w1105, "Read Timeout (ms)"=u32 2000, "GEA Inputs"=w1107, "Write ERD List"=w1110, "Error In"=w1111, "Verify ERD Response?"=FALSE) -> ("GEA2 Reference Out"=w1104:refnum<k24>, "Error Out"=w1103:errorcluster)  [unwired: 7 in, 1 out]
          }
          event "Lid Lock.Lock Lid", "Lid Lock.Unlock Lid": Value Change {
            n80 = event-data() -> ("CtlRef"=w1118:refnum<vi>)  [unwired: 1 in, 5 out]
            n81 = property class="Bool"(reference=w1118, error in=w1121) -> (reference out=w1124:refnum<vi>, error out=w1125:errorcluster, "Label.Text"=w1126:string)
            n82 = Close Reference(reference=w1124, error in (no error)=w1125) -> (error out=w1123:errorcluster)
            n83 = case shown="\"Unlock Lid\", Default" w1126 {
              tunnel: [w1131 w1157] -> _
              tunnel: w1120 -> [w1132 w1156]
              tunnel: w1123 -> [w1133 w1148]
              tunnel: w1119 -> [w1130 w1147]
              tunnel: [w1129 w1146] -> _
              tunnel: T24 {"ERD Number"=61441, "Data Type"=enum."string", "Data"=""} ("ERD Read Data In") -> [w1127 w1144]
              frame "Unlock Lid", Default {
                n84 = Concatenate Strings("00" ("string")) -> (w1143:string)
                n85 = Bundle By Name(cluster=w1127, "Data"=w1143) -> (w1142:T24)
                n86 = Build Array(w1142) -> (w1135:T24[])
                n87 = call "Convert Write ERD List to Message.vi"("GEA Inputs"=w1130, "Write ERD List"=w1135, "Error In"=w1133) -> ("GEA Message"=w1137:T3, "Error Out"=w1138:errorcluster)  [unwired: 11 in]
                n88 = call "GEA2MessageFormatter.vi"("Prefix(Send/Recv)"="SEND", "GEA2 Data In"=w1137, "Error In"=w1138) -> ("Output String"=w1139:string, "Error Out"=w1140:errorcluster)  [unwired: 11 in]
                n89 = call "GExplorer_Queue_GEA2.vi"("Output String"=w1139, "error in (no error)"=w1140) -> ("error out"=w1136:errorcluster)  [unwired: 13 in]
                n90 = call "GEA2 Write ERD.vi"("GEA2 Reference In"=w1132, "GEA Inputs"=w1130, "Write ERD List"=w1135, "Error In"=w1136, "Verify ERD Response?"=FALSE) -> ("GEA2 Reference Out"=w1129:refnum<k24>, "Error Out"=w1131:errorcluster)  [unwired: 8 in, 1 out]
              }
              frame "Lock Lid" {
                n91 = Concatenate Strings("01" ("string")) -> (w1160:string)
                n92 = Bundle By Name(cluster=w1144, "Data"=w1160) -> (w1159:T24)
                n93 = Build Array(w1159) -> (w1150:T24[])
                n94 = call "Convert Write ERD List to Message.vi"("GEA Inputs"=w1147, "Write ERD List"=w1150, "Error In"=w1148) -> ("GEA Message"=w1152:T3, "Error Out"=w1153:errorcluster)  [unwired: 11 in]
                n95 = call "GEA2MessageFormatter.vi"("Prefix(Send/Recv)"="SEND", "GEA2 Data In"=w1152, "Error In"=w1153) -> ("Output String"=w1154:string, "Error Out"=w1155:errorcluster)  [unwired: 11 in]
                n96 = call "GExplorer_Queue_GEA2.vi"("Output String"=w1154, "error in (no error)"=w1155) -> ("error out"=w1151:errorcluster)  [unwired: 13 in]
                n97 = call "GEA2 Write ERD.vi"("GEA2 Reference In"=w1156, "GEA Inputs"=w1147, "Write ERD List"=w1150, "Error In"=w1151, "Verify ERD Response?"=FALSE) -> ("GEA2 Reference Out"=w1146:refnum<k24>, "Error Out"=w1157:errorcluster)  [unwired: 8 in, 1 out]
              }
            }
          }
          event "Test Mode.Exit", "Test Mode.Enter": Value Change {
            n98 = event-data() -> ("CtlRef"=w1161:refnum<vi>)  [unwired: 1 in, 5 out]
            n99 = property class="Bool"(reference=w1161, error in=w1164) -> (reference out=w1167:refnum<vi>, error out=w1168:errorcluster, "Label.Text"=w1169:string)
            n100 = Close Reference(reference=w1167, error in (no error)=w1168) -> (error out=w1166:errorcluster)
            n101 = case shown="\"Exit\"" w1169 {
              tunnel: [w1174 w1200] -> _
              tunnel: w1163 -> [w1175 w1199]
              tunnel: w1166 -> [w1176 w1191]
              tunnel: w1162 -> [w1173 w1190]
              tunnel: [w1172 w1189] -> _
              tunnel: T24 {"ERD Number"=61440, "Data Type"=enum."string", "Data"=""} ("ERD Read Data In") -> [w1170 w1187]
              frame "Enter", Default {
                n102 = Concatenate Strings("01" ("string")) -> (w1186:string)
                n103 = Bundle By Name(cluster=w1170, "Data"=w1186) -> (w1185:T24)
                n104 = Build Array(w1185) -> (w1178:T24[])
                n105 = call "Convert Write ERD List to Message.vi"("GEA Inputs"=w1173, "Write ERD List"=w1178, "Error In"=w1176) -> ("GEA Message"=w1180:T3, "Error Out"=w1181:errorcluster)  [unwired: 11 in]
                n106 = call "GEA2MessageFormatter.vi"("Prefix(Send/Recv)"="SEND", "GEA2 Data In"=w1180, "Error In"=w1181) -> ("Output String"=w1182:string, "Error Out"=w1183:errorcluster)  [unwired: 11 in]
                n107 = call "GExplorer_Queue_GEA2.vi"("Output String"=w1182, "error in (no error)"=w1183) -> ("error out"=w1179:errorcluster)  [unwired: 13 in]
                n108 = call "GEA2 Write ERD.vi"("GEA2 Reference In"=w1175, "GEA Inputs"=w1173, "Write ERD List"=w1178, "Error In"=w1179, "Verify ERD Response?"=FALSE) -> ("GEA2 Reference Out"=w1172:refnum<k24>, "Error Out"=w1174:errorcluster)  [unwired: 8 in, 1 out]
              }
              frame "Exit" {
                n109 = Concatenate Strings("00" ("string")) -> (w1203:string)
                n110 = Bundle By Name(cluster=w1187, "Data"=w1203) -> (w1202:T24)
                n111 = Build Array(w1202) -> (w1193:T24[])
                n112 = call "Convert Write ERD List to Message.vi"("GEA Inputs"=w1190, "Write ERD List"=w1193, "Error In"=w1191) -> ("GEA Message"=w1195:T3, "Error Out"=w1196:errorcluster)  [unwired: 11 in]
                n113 = call "GEA2MessageFormatter.vi"("Prefix(Send/Recv)"="SEND", "GEA2 Data In"=w1195, "Error In"=w1196) -> ("Output String"=w1197:string, "Error Out"=w1198:errorcluster)  [unwired: 11 in]
                n114 = call "GExplorer_Queue_GEA2.vi"("Output String"=w1197, "error in (no error)"=w1198) -> ("error out"=w1194:errorcluster)  [unwired: 13 in]
                n115 = call "GEA2 Write ERD.vi"("GEA2 Reference In"=w1199, "GEA Inputs"=w1190, "Write ERD List"=w1193, "Error In"=w1194, "Verify ERD Response?"=FALSE) -> ("GEA2 Reference Out"=w1189:refnum<k24>, "Error Out"=w1200:errorcluster)  [unwired: 8 in, 1 out]
              }
            }
          }
          event "Clear Fault Table Buffer": Value Change {
            n116 = event-data() -> ()  [unwired: 1 in, 6 out]
            n117 = Bundle By Name(cluster=T24 {"ERD Number"=130, "Data Type"=enum."string", "Data"=""} ("ERD Read Data In"), "Data"="FF") -> (w1219:T24)
            n118 = Build Array(w1219) -> (w1213:T24[])
            n119 = call "Convert Write ERD List to Message.vi"("GEA Inputs"=w1210, "Write ERD List"=w1213, "Error In"=w1209) -> ("GEA Message"=w1215:T3, "Error Out"=w1216:errorcluster)  [unwired: 11 in]
            n120 = call "GEA2MessageFormatter.vi"("Prefix(Send/Recv)"="SEND", "GEA2 Data In"=w1215, "Error In"=w1216) -> ("Output String"=w1217:string, "Error Out"=w1218:errorcluster)  [unwired: 11 in]
            n121 = call "GExplorer_Queue_GEA2.vi"("Output String"=w1217, "error in (no error)"=w1218) -> ("error out"=w1214:errorcluster)  [unwired: 13 in]
            n122 = call "GEA2 Write ERD.vi"("GEA2 Reference In"=w1208, "Read Timeout (ms)"=u32 2000, "GEA Inputs"=w1210, "Write ERD List"=w1213, "Error In"=w1214, "Verify ERD Response?"=FALSE) -> ("GEA2 Reference Out"=w1207:refnum<k24>, "Error Out"=w1206:errorcluster)  [unwired: 7 in, 1 out]
          }
          event "Clear Cycle Buffer": Value Change {
            n123 = event-data() -> ()  [unwired: 1 in, 6 out]
            n124 = Build Array(T24 {"ERD Number"=136, "Data Type"=enum."string", "Data"="FF"} ("ERD Read Data In")) -> (w1233:T24[])
            n125 = call "Convert Write ERD List to Message.vi"("GEA Inputs"=w1228, "Write ERD List"=w1233, "Error In"=w1231) -> ("GEA Message"=w1235:T3, "Error Out"=w1236:errorcluster)  [unwired: 11 in]
            n126 = call "GEA2MessageFormatter.vi"("Prefix(Send/Recv)"="SEND", "GEA2 Data In"=w1235, "Error In"=w1236) -> ("Output String"=w1237:string, "Error Out"=w1238:errorcluster)  [unwired: 11 in]
            n127 = call "GExplorer_Queue_GEA2.vi"("Output String"=w1237, "error in (no error)"=w1238) -> ("error out"=w1234:errorcluster)  [unwired: 13 in]
            n128 = call "GEA2 Write ERD.vi"("GEA2 Reference In"=w1230, "GEA Inputs"=w1228, "Write ERD List"=w1233, "Error In"=w1234) -> ("Error Out"=w1227:errorcluster)  [unwired: 9 in, 2 out]
            n129 = call "Time Delay6"("error in (no error)"=w1227) -> ("error out"=w1222:errorcluster)  [unwired: 10 in]
            n130 = property on="Get Cycle History" class="Bool (strict)"(error in=w1222, "Val(Sgnl)"=TRUE ("Get Cycle History")) -> (error out=w1226:errorcluster)  [unwired: 1 in, 1 out]
            n131 = call "Time Delay7"("error in (no error)"=w1226) -> ("error out"=w1221:errorcluster)  [unwired: 10 in]
            n132 = property on="Get Cycle History" class="Bool (strict)"(error in=w1221, "Val(Sgnl)"=FALSE ("Get Cycle History")) -> (error out=w1225:errorcluster)  [unwired: 1 in, 1 out]
          }
          event "Get Cycle History": Value Change {
            w1245 = T6[] [{"ERD Number"=135, "Data Type"=enum."string"}, {"ERD Number"=57344, "Data Type"=enum."string"}, {"ERD Number"=57345, "Data Type"=enum."string"}, {"ERD Number"=57346, "Data Type"=enum."string"}, {"ERD Number"=57347, "Data Type"=enum."string"}, {"ERD Number"=57348, "Data Type"=enum."string"}, {"ERD Number"=57349, "Data Type"=enum."string"}, {"ERD Number"=57350, "Data Type"=enum."string"}, {"ERD Number"=57351, "Data Type"=enum."string"}, {"ERD Number"=57352, "Data Type"=enum."string"}, {"ERD Number"=57353, "Data Type"=enum."string"}] ("Read ERD List")
            n133 = event-data() -> ()  [unwired: 1 in, 6 out]
            n134 = call "Convert Read ERD List to Message.vi"("GEA Inputs"=w1240, "Read ERD List"=w1245, "Error In"=w1247) -> ("GEA Message"=w1251:T3, "Error Out"=w1252:errorcluster)  [unwired: 11 in]
            n135 = call "GEA2MessageFormatter.vi"("Prefix(Send/Recv)"="SEND", "GEA2 Data In"=w1251, "Error In"=w1252) -> ("Output String"=w1250:string, "Error Out"=w1249:errorcluster)  [unwired: 11 in]
            n136 = call "GExplorer_Queue_GEA2.vi"("Output String"=w1250, "error in (no error)"=w1249) -> ("error out"=w1246:errorcluster)  [unwired: 13 in]
            n137 = call "GEA2 Read ERD Multiple Messages.vi"("GEA2 Reference In"=w1241, "Read Timeout (ms)"=u32 500, "GEA Inputs"=w1240, "Read ERD List"=w1245, "Error In"=w1246, "#ERDs per message"=4, "Verify ERD Response?"=TRUE) -> ("ERD Data Out"=w1253:T30[], "Error Out"=w1244:errorcluster)  [unwired: 5 in, 2 out]
            n138 = call "Cycle_Diag_Table_Read_TL24.vi"("ERD Data In"=w1253, "error in (no error)"=w1244) -> ("Cycle Buffer Status"=→"Cycle Buffer Status":T14, "Diag Cycle String Out"=→"Diagnostics Table":string[][], "error out"=w1239:errorcluster)  [unwired: 10 in, 1 out]
          }
          event "Save Cycle History Log": Value Change {
            w1261 = T6[] [{"ERD Number"=135, "Data Type"=enum."string"}, {"ERD Number"=57344, "Data Type"=enum."string"}, {"ERD Number"=57345, "Data Type"=enum."string"}, {"ERD Number"=57346, "Data Type"=enum."string"}, {"ERD Number"=57347, "Data Type"=enum."string"}, {"ERD Number"=57348, "Data Type"=enum."string"}, {"ERD Number"=57349, "Data Type"=enum."string"}, {"ERD Number"=57350, "Data Type"=enum."string"}, {"ERD Number"=57351, "Data Type"=enum."string"}, {"ERD Number"=57352, "Data Type"=enum."string"}, {"ERD Number"=57353, "Data Type"=enum."string"}] ("Read ERD List")
            n139 = event-data() -> ()  [unwired: 1 in, 6 out]
            n140 = call "Convert Read ERD List to Message.vi"("GEA Inputs"=w1264, "Read ERD List"=w1261, "Error In"=w1263) -> ("GEA Message"=w1270:T3, "Error Out"=w1271:errorcluster)  [unwired: 11 in]
            n141 = call "GEA2MessageFormatter.vi"("Prefix(Send/Recv)"="SEND", "GEA2 Data In"=w1270, "Error In"=w1271) -> ("Output String"=w1269:string, "Error Out"=w1268:errorcluster)  [unwired: 11 in]
            n142 = call "GExplorer_Queue_GEA2.vi"("Output String"=w1269, "error in (no error)"=w1268) -> ("error out"=w1266:errorcluster)  [unwired: 13 in]
            n143 = call "GEA2 Read ERD Multiple Messages.vi"("GEA2 Reference In"=w1262, "Read Timeout (ms)"=u32 500, "GEA Inputs"=w1264, "Read ERD List"=w1261, "Error In"=w1266, "#ERDs per message"=4, "Verify ERD Response?"=TRUE) -> ("ERD Data Out"=w1260:T30[], "Error Out"=w1265:errorcluster)  [unwired: 5 in, 2 out]
            n144 = call "Cycle_Diag_Table_Read_TL24.vi"("ERD Data In"=w1260, "error in (no error)"=w1265) -> ("Diag Cycle String Out"=w1259:string[][], "error out"=w1258:errorcluster)  [unwired: 10 in, 2 out]
            n145 = call "Cycle_History_Logging.vi"("error in (no error)"=w1258, "Diag Cycle String Out"=w1259) -> ("error out"=w1257:errorcluster)  [unwired: 9 in]
          }
          event "Data ON": Value Change {
            n146 = event-data() -> ()  [unwired: 1 in, 6 out]
            n147 = case shown="True" "Data ON" {
              tunnel: w1278 -> [w1281 w1285]
              tunnel: [w1280 w1284] -> w1277
              tunnel: w1275 -> [w1279 w1283]
              frame True {
                n148 = Enqueue Element(queue=w1279, element=T21 {"Data"=variant, "State"=enum."Init"} ("Data"), error in (no error)=w1281) -> (error out=w1280:errorcluster)  [unwired: 1 in, 2 out]
              }
              frame False {
                n149 = Enqueue Element(queue=w1283, element=T21 {"Data"=variant, "State"=enum."Pause"} ("Data"), error in (no error)=w1285) -> (error out=w1284:errorcluster)  [unwired: 1 in, 2 out]
              }
            }
          }
          event "Stop": Value Change; User Event; Panel Close {
            n150 = event-data() -> ()  [unwired: 1 in, 3 out]
            n151 = call "Control_ERD_Loop_Brass.vi"("Command (ERD Loop Control)"=ERD_Loop_Control_Command_Brass."Shutdown", "Error In"=w1295) -> ("Error Out"=w1294:errorcluster)  [unwired: 13 in]
            n152 = call "Control_GEA2_Loop_Brass.vi"("Command (ERD Loop Control)"=GEA2_Control_Command_Brass."Shutdown", "Error In"=w1294) -> ("Error Out"=w1296:errorcluster)  [unwired: 13 in]
            n153 = call "Control_DAQ_Loop_Brass.vi"("Command (DAQ Control)"=DAQ_Control_Command_Brass."Shutdown", "Error In"=w1296) -> ("Error Out"=w1299:errorcluster)  [unwired: 13 in]
            n154 = call "Control_Cont_Send_Brass.vi"("Command (ERD Loop Control)"=GEA2_Control_Command_Brass."Shutdown", "Error In"=w1299) -> ("Error Out"=w1289:errorcluster)  [unwired: 13 in]
            n155 = call "Time Delay8"("error in (no error)"=w1289, "Delay Time (s)"=2.0) -> ("error out"=w1288:errorcluster)  [unwired: 9 in]
          }
        }
        n156 = call "Error_Control_Brass.vi"("Error In"=w1010) -> ("Error Out"=w1012:errorcluster)  [unwired: 14 in]
      }
      n157 = Unbundle By Name(T21 {"Data"=variant, "State"=enum."Init"} ("Data")) -> ("State"=w68:T22)
      n158 = Build Array(w22, w63, w61, w62) -> (w60:refnum<vi>[])
      n159 = while "DAQ Loop" {
        shift-right: [w485] -> w95
        shift-left: w32 -> [w483]
        shift-right: [w462] -> _
        shift-left: DAQ_States_Brass."Wait for Init" ("States") -> [w480]
        shift-right: [w463] -> _
        shift-left: "Wait for Init" ("Report Text") -> [w478]
        tunnel: w59 -> [w479]
        shift-right: [w461] -> _
        shift-left: _ -> [w418]
        shift-right: [w460] -> _
        shift-left: FALSE -> [w459]
        shift-right: [w449] -> _
        shift-left: w51 -> [w448]
        shift-right: [w447] -> _
        shift-left: w51 -> [w446]
        shift-right: [w445] -> _
        shift-left: w51 -> [w444]
        shift-right: [w443] -> _
        shift-left: w51 -> [w442]
        shift-right: [w441] -> _
        shift-left: w51 -> [w440]
        shift-right: [w439] -> _
        shift-left: w51 -> [w438]
        shift-right: [w437] -> _
        shift-left: w51 -> [w436]
        shift-right: [w423] -> _
        shift-left: 1.0 -> [w419]
        shift-right: [w422] -> _
        shift-left: 1.0 -> [w426]
        shift-right: [w421] -> _
        shift-left: 0.0 -> [w425]
        shift-right: [w417] -> _
        shift-left: w51 -> [w416]
        shift-right: [w415] -> _
        shift-left: FALSE -> [w450]
        stop <- w475 stop-if-true
        # "Automatic Modeshift Feedback"
        # "DAQ Loop"
        n160 = Greater?(x=w426, y=5.0 ("x")) -> (0:w428:bool)
        n161 = Dequeue Element(queue=w479, timeout in ms (-1)=0, error in (no error)=w483) -> (element=w481:T20, timed out?=w482:bool, error out=w474:errorcluster)  [unwired: 1 out]
        n162 = Wait (ms)(milliseconds to wait=u32 250) -> ()  [unwired: 1 out]
        n163 = Select(t="Basket RPM", s=w428, f=w419) -> (s? t:f=w423:dbl)
        n164 = Select(t=w480, s=w482, f=w481) -> (s? t:f=w477:T20)
        n165 = Multiply(x=w423, y=0.40625) -> (x*y=w454:dbl)
        n166 = Less?(x=w423, y=1.0) -> (x < y?=w452:bool)
        n167 = Equal?(x=w419, y=w423) -> (x = y?=w451:bool)
        n168 = case shown="\"Run\"" w477 {
          selector: w477 -> [_ _ _ _ _ _ w964]
          tunnel: [_ _ _ w677 w797 _ _] -> w417
          tunnel: [w517 w541 w573 w678 w795 w902 w967] -> w471
          tunnel: w436 -> [w532 w556 w581 _ w794 w896 w913]
          tunnel: [w532 w556 w581 w682 w793 _ _] -> w437
          tunnel: w438 -> [w531 w555 w582 _ w792 w893 w940]
          tunnel: [w531 w555 w582 w686 w791 _ _] -> w439
          tunnel: [w515 w539 w565 w685 w790 w856 w930] -> w469
          tunnel: [w516 w540 w566 w681 w789 w863 w942] -> w470
          tunnel: [w526 DAQ_States_Brass."Verify Hardware" ("t") w578 DAQ_States_Brass."Run" ("t") w767 DAQ_States_Brass."Wait for Init" ("States") w964] -> w462
          tunnel: [FALSE FALSE FALSE TRUE TRUE FALSE FALSE] -> w461
          tunnel: w444 -> [w530 w554 w585 _ w752 w900 w969]
          tunnel: [w512 w536 w562 w674 w786 w849 w927] -> w466
          tunnel: [w530 w554 w585 w675 w787 _ _] -> w445
          tunnel: [w513 w537 w563 w638 w777 w888 w968] -> w467
          tunnel: w442 -> [w529 w553 w584 _ w776 w899 w963]
          tunnel: [w529 w553 w584 w643 w778 _ _] -> w443
          tunnel: [_ _ _ _ _ FALSE TRUE] -> w475
          tunnel: [_ _ _ _ w785 _ _] -> w435
          tunnel: [_ _ _ _ w779 _ _] -> w420
          tunnel: [_ _ _ _ w784 _ _] -> w434
          tunnel: [_ _ _ _ w783 _ _] -> w433
          tunnel: [_ _ _ _ w782 _ _] -> w432
          tunnel: [_ _ _ _ w781 _ _] -> w431
          tunnel: [_ _ _ _ w780 _ _] -> w430
          tunnel: [w514 w538 w564 w635 w775 w886 w961] -> w468
          tunnel: [w528 w552 w583 w632 w773 _ _] -> w441
          tunnel: w440 -> [w528 w552 w583 _ w774 w887 w962]
          tunnel: [_ _ _ _ w772 _ _] -> w458
          tunnel: [_ _ _ _ w771 _ _] -> w457
          tunnel: [w527 w551 w575 "Initialize" ("Report Text") "Running" ("Report Text") "Wait for Init" ("Report Text") "Exit" ("Report Text")] -> w463
          tunnel: w478 -> [w527 w551 _ _ _ _ _]
          tunnel: [w511 w535 w561 w616 w759 w880 w958] -> w465
          tunnel: [w522 w549 w571 w613 w758 _ _] -> w447
          tunnel: [w521 w548 w570 w611 w756 _ _] -> w449
          tunnel: [w510 w534 w560 w610 w757 w879 w905] -> w464
          tunnel: w446 -> [w522 w549 w571 _ w760 w881 w959]
          tunnel: w448 -> [w521 w548 w570 _ w755 w877 w925]
          tunnel: [w509 w533 w559 w590 w754 FALSE FALSE] -> w460
          tunnel: [FALSE FALSE FALSE FALSE w744 FALSE FALSE] -> w415
          tunnel: [w518 w544 w568 w597 w743 w872 w955] -> w472
          tunnel: "Turn On DAQ" -> [w519 _ _ _ w719 _ _]
          tunnel: w474 -> [w517 w541 w567 w599 w742 w871 w954]
          tunnel: w474 -> [w516 w540 w566 w598 w737 w869 w916]
          tunnel: w474 -> [w518 w543 w568 w597 w743 w872 w955]
          tunnel: w474 -> [w515 w539 w565 w596 w735 w854 w939]
          tunnel: w474 -> [w514 w538 w564 w595 w734 w853 w953]
          tunnel: w474 -> [w513 w537 w563 w594 w731 w852 w952]
          tunnel: w474 -> [w512 w536 w562 w593 w730 w851 w951]
          tunnel: w474 -> [w511 w535 w561 w592 w724 w847 w950]
          tunnel: w474 -> [w510 w534 w560 w591 w720 w846 w924]
          tunnel: w459 -> [w509 w533 w559 w590 w723 _ _]
          tunnel: w454 -> [_ _ _ _ w729 _ _]
          tunnel: 0.5 ("Duty Cycle") -> [_ _ _ _ w728 _ _]
          tunnel: w452 -> [_ _ _ _ w726 _ _]
          tunnel: w451 -> [_ _ _ _ w727 _ _]
          tunnel: w450 -> [_ _ _ _ w725 _ _]
          tunnel: w418 -> [_ _ _ _ _ _ w949]
          tunnel: w416 -> [_ _ _ _ w718 w845 w948]
          frame "Wait for Init", Default {
            # "Hall Sensor"
            # "Motor TRIAC CCW"
            # "Motor TRIAC CW"
            # "Relay Controls"
            # "TRIAC Outputs"
            # "AO for ADC"
            n169 = Select(t=DAQ_States_Brass."Rename Devices", s=w519, f=DAQ_States_Brass."Wait for Init" ("States")) -> (s? t:f=w526:T20)
          }
          frame "Rename Devices" {
            # "Hall Sensor"
            # "Motor TRIAC CCW"
            # "Motor TRIAC CW"
            # "Relay Controls"
            # "TRIAC Outputs"
            n170 = case shown="\"LE\"" "HE/LE ?" {
              tunnel: ["VALEW_HE" "VALEW_LE"] -> w545
              frame "HE", Default {
              }
              frame "LE" {
              }
            }
            n171 = call "VALEW_Rename DAQmx Devices.vi"("cDAQ Name"=w545, "Error In"=w543) -> ("Error Out"=w544:errorcluster)  [unwired: 13 in]
          }
          frame "Verify Hardware" {
            n172 = call "DeviceListCheck.vi"("Device List"=string[] ["9481_1", "9435_1", "9435_2", "9401_1", "9269_1"], "Error In"=w567) -> ("Devices Present?"=w572:bool, "Report Text"=w575:string, "Error Out"=w574:errorcluster)  [unwired: 11 in]
            n173 = case shown="False" w572 {
              selector: w572 -> [w587 _]
              tunnel: w574 -> [w588 w589]
              tunnel: [w586 w589] -> w573
              frame False {
                n174 = property on="Turn On DAQ" class="Bool (strict)"(error in=w588, "Value"=w587) -> (error out=w586:errorcluster)  [unwired: 1 in, 1 out]
              }
              frame True {
              }
            }
            n175 = Select(t=DAQ_States_Brass."Initialize" ("f"), s=w572, f=DAQ_States_Brass."Wait for Init") -> (s? t:f=w578:T20)
          }
          frame "Initialize" {
            w604 = 4 items=["verify"=2, "reserve"=4, "commit"=3, "unreserve"=5, "abort"=6] ("action")
            w620 = 10123 items=["Finite Samples"=10178, "Continuous Samples"=10123, "Hardware Timed Single Point"=12522] ("sample mode")
            w623 = 4 items=["verify"=2, "reserve"=4, "commit"=3, "unreserve"=5, "abort"=6] ("action")
            w656 = 4 items=["verify"=2, "reserve"=4, "commit"=3, "unreserve"=5, "abort"=6] ("action")
            w657 = 4 items=["verify"=2, "reserve"=4, "commit"=3, "unreserve"=5, "abort"=6] ("action")
            w671 = 10123 items=["Finite Samples"=10178, "Continuous Samples"=10123, "Hardware Timed Single Point"=12522] ("sample mode")
            w679 = 0 items=["one channel for each line", "one channel for all lines"] ("line grouping")
            w684 = 0 items=["one channel for each line", "one channel for all lines"] ("line grouping")
            w687 = 0.0  # minimum value
            w688 = 5.0  # maximum value
            # "Hall Sensor"
            # "Motor TRIAC CCW"
            # "Motor TRIAC CW"
            # "Relay Controls"
            # "TRIAC Outputs"
            # "AO for ADC"
            n176 = call <vilib>:"DAQmx Create Task.vi"("auto cleanup"=TRUE, "error in"=w593) -> ("task out"=w645:refnum<k21>, "error out"=w646:errorcluster)  [unwired: 12 in]
            n177 = call <vilib>:"DAQmx Create Task.vi"("auto cleanup"=TRUE, "error in"=w592) -> ("task out"=w619:refnum<k21>, "error out"=w618:errorcluster)  [unwired: 12 in]
            n178 = call <vilib>:"DAQmx Create Task.vi"("auto cleanup"=TRUE, "error in"=w595) -> ("task out"=w653:refnum<k21>, "error out"=w654:errorcluster)  [unwired: 12 in]
            n179 = call <vilib>:"DAQmx Create Task.vi"("auto cleanup"=TRUE, "error in"=w594) -> ("task out"=w651:refnum<k21>, "error out"=w652:errorcluster)  [unwired: 12 in]
            n180 = call-poly <vilib>:"DAQmx Create Virtual Channel.vi"("task in"=w645, "counter"=tag "9401_1/ctr2", "error in"=w646) -> ("task out"=w648:refnum<k21>, "error out"=w676:errorcluster)  [unwired: 11 in]
            n181 = call-poly <vilib>:"DAQmx Create Virtual Channel.vi"("task in"=w653, "counter"=tag "9401_1/ctr0", "error in"=w654) -> ("task out"=w666:refnum<k21>, "error out"=w662:errorcluster)  [unwired: 11 in]
            n182 = call-poly <vilib>:"DAQmx Create Virtual Channel.vi"("task in"=w651, "counter"=tag "9401_1/ctr1", "error in"=w652) -> ("task out"=w665:refnum<k21>, "error out"=w664:errorcluster)  [unwired: 11 in]
            n183 = call-poly <vilib>:"DAQmx Create Virtual Channel.vi"("task in"=w619, "lines"=tag "9401_1/port0/line2", "error in"=w618) -> ("task out"=w625:refnum<k21>, "error out"=w626:errorcluster)  [unwired: 11 in]
            n184 = property class="DAQmx Channel"(reference=w648, error in=w676, "CO.Pulse.Term"=tag "/9401_1/PFI4") -> (reference out=w673:refnum<k21>, error out=w672:errorcluster)
            n185 = call-poly <vilib>:"DAQmx Create Virtual Channel.vi"("lines"=tag "9481_1/port0/line3", "error in"=w591) -> ("task out"=w611:refnum<k21>, "error out"=w610:errorcluster)  [unwired: 12 in]
            n186 = property class="DAQmx Channel"(reference=w666, error in=w662, "CI.CountEdges.Term"=tag "/9401_1/PFI0") -> (reference out=w661:refnum<k21>, error out=w660:errorcluster)
            n187 = property class="DAQmx Channel"(reference=w665, error in=w664, "CI.CountEdges.Term"=tag "/9401_1/PFI1") -> (reference out=w659:refnum<k21>, error out=w658:errorcluster)
            n188 = call-poly <vilib>:"DAQmx Create Virtual Channel.vi"("lines"=tag "9481_1/port0/line0:2", "name to assign"="Relay Outputs", "line grouping"=w684, "error in"=w598) -> ("task out"=w682:refnum<k21>, "error out"=w681:errorcluster)  [unwired: 10 in]
            n189 = call-poly <vilib>:"DAQmx Create Virtual Channel.vi"("lines"=tag "9435_1/port0/line0:2, 9435_2/port0/line0:3", "name to assign"="Outputs", "line grouping"=w679, "error in"=w599) -> ("task out"=w677:refnum<k21>, "error out"=w678:errorcluster)  [unwired: 10 in]
            n190 = call-poly <vilib>:"DAQmx Create Virtual Channel.vi"("maximum value"=w688, "minimum value"=w687, "physical channels"=tag "9269_1/ao0:2" ("lines"), "name to assign"="AO for ADC", "error in"=w596) -> ("task out"=w686:refnum<k21>, "error out"=w685:errorcluster)  [unwired: 9 in]
            n191 = call-poly <vilib>:"DAQmx Timing.vi"("task/channels in"=w625, "sample mode"=w620, "rate"=1000.0, "error in"=w626) -> ("task out"=w621:refnum<k21>, "error out"=w622:errorcluster)  [unwired: 10 in]
            n192 = call-poly <vilib>:"DAQmx Timing.vi"("task/channels in"=w673, "sample mode"=w671, "error in"=w672) -> ("task out"=w603:refnum<k21>, "error out"=w600:errorcluster)  [unwired: 11 in]
            n193 = call <vilib>:"DAQmx Control Task.vi"("task/channels in"=w661, "action"=w656, "error in"=w660) -> ("task out"=w634:refnum<k21>, "error out"=w637:errorcluster)  [unwired: 11 in]
            n194 = call <vilib>:"DAQmx Control Task.vi"("task/channels in"=w659, "action"=w657, "error in"=w658) -> ("task out"=w642:refnum<k21>, "error out"=w640:errorcluster)  [unwired: 11 in]
            n195 = call <vilib>:"DAQmx Control Task.vi"("task/channels in"=w603, "action"=w604, "error in"=w600) -> ("task out"=w602:refnum<k21>, "error out"=w601:errorcluster)  [unwired: 11 in]
            n196 = call <vilib>:"DAQmx Control Task.vi"("task/channels in"=w621, "action"=w623, "error in"=w622) -> ("task out"=w614:refnum<k21>, "error out"=w615:errorcluster)  [unwired: 11 in]
            n197 = flat-sequence {
              tunnel: w602 -> [w692]
              tunnel: w601 -> [w691]
              tunnel: w642 -> [w700]
              tunnel: [w700] -> w641
              tunnel: w640 -> [w699]
              tunnel: [w699] -> w639
              tunnel: w637 -> [w698]
              tunnel: [w698] -> w636
              tunnel: w634 -> [w697]
              tunnel: [w697] -> w633
              tunnel: w615 -> [w695]
              tunnel: w614 -> [w696]
              tunnel: [w694] -> w608
              tunnel: [w693] -> w607
              tunnel: [w692] -> w606
              tunnel: [w691] -> w605
              tunnel: [w704] -> w674
              tunnel: [w703] -> w675
              tunnel: [w714] -> w643
              tunnel: w641 -> [w713]
              tunnel: w639 -> [w712]
              tunnel: [w711] -> w638
              tunnel: w636 -> [w710]
              tunnel: [w709] -> w635
              tunnel: w633 -> [w708]
              tunnel: [w707] -> w632
              tunnel: [w706] -> w616
              tunnel: [w705] -> w613
              tunnel: w608 -> [w706]
              tunnel: w607 -> [w705]
              tunnel: w606 -> [w702]
              tunnel: w605 -> [w701]
              frame #0 {
                n198 = call <vilib>:"DAQmx Start Task.vi"("task/channels in"=w696, "error in"=w695) -> ("task out"=w693:refnum<k21>, "error out"=w694:errorcluster)  [unwired: 12 in]
              }
              frame #1 {
                n199 = call <vilib>:"DAQmx Start Task.vi"("task/channels in"=w708, "error in"=w710) -> ("task out"=w707:refnum<k21>, "error out"=w709:errorcluster)  [unwired: 12 in]
                n200 = call <vilib>:"DAQmx Start Task.vi"("task/channels in"=w713, "error in"=w712) -> ("task out"=w714:refnum<k21>, "error out"=w711:errorcluster)  [unwired: 12 in]
                n201 = call <vilib>:"DAQmx Start Task.vi"("task/channels in"=w702, "error in"=w701) -> ("task out"=w703:refnum<k21>, "error out"=w704:errorcluster)  [unwired: 12 in]
              }
            }
          }
          frame "Run" {
            # "Lid Lock Feedback"
            # "Is the task stopped?"
            # "Hall Sensor"
            # "Motor TRIAC CCW"
            # "Motor TRIAC CW"
            # "AO for ADC"
            # "Relay Controls"
            # "TRIAC Outputs"
            n202 = case shown="True" w726 {
              tunnel: w752 -> [w831 w836]
              tunnel: [w831 w835] -> w750
              tunnel: [w830 w834] -> w751
              tunnel: [w829 TRUE] -> w745
              tunnel: w730 -> [w830 w832]
              tunnel: w725 -> [w829 _]
              frame False {
              }
              frame True {
                n203 = call <vilib>:"DAQmx Stop Task.vi"("task/channels in"=w836, "error in"=w832) -> ("task out"=w835:refnum<k21>, "error out"=w834:errorcluster)  [unwired: 12 in]
              }
            }
            n204 = call-poly <vilib>:"DAQmx Read.vi"("task/channels in"=w760, "number of samples per channel"=-1, "timeout"=10.0, "error in"=w724) -> ("task out"=w758:refnum<k21>, "data"=w764:u8[], "error out"=w759:errorcluster)  [unwired: 9 in]
            n205 = Compound Arithmetic op=AND(w745, invert w726) -> (w747:bool)
            n206 = case shown="False" w747 {
              tunnel: w751 -> [w821 w825]
              tunnel: w750 -> [w822 w824]
              tunnel: [w822 w828] -> w749
              tunnel: [w821 w827] -> w748
              tunnel: w745 -> [w820 _]
              tunnel: [w820 FALSE] -> w744
              frame False {
              }
              frame True {
                n207 = call <vilib>:"DAQmx Start Task.vi"("task/channels in"=w824, "error in"=w825) -> ("task out"=w828:refnum<k21>, "error out"=w827:errorcluster)  [unwired: 12 in]
                n208 = Wait (ms)(milliseconds to wait=u32 1200) -> ()  [unwired: 1 out]
              }
            }
            n209 = Build Array("AC Power", "Mode Shift FB", "Lid Status") -> (w738:bool[])
            n210 = Build Array("Pressure", "Motor Current", "Temperature") -> (w736:dbl[])
            n211 = Search 1D Array(1D array=w764, element=u8 4) -> (index of element=w762:i32)  [unwired: 1 in]
            n212 = Equal?(x=w762, y=-1) -> (x = y?=w753:bool)
            n213 = Compound Arithmetic op=OR(w726, w727) -> (w746:bool)
            n214 = call-poly <vilib>:"DAQmx Read.vi"("task/channels in"=w718, "error in"=w742) -> ("task out"=w797:refnum<k21>, "data"=w796:bool[], "error out"=w795:errorcluster)  [unwired: 11 in]
            n215 = call-poly <vilib>:"DAQmx Write.vi"("task/channels in"=w794, "data"=w738, "error in"=w737) -> ("task out"=w793:refnum<k21>, "error out"=w789:errorcluster)  [unwired: 10 in, 1 out]
            n216 = call-poly <vilib>:"DAQmx Write.vi"("task/channels in"=w792, "data"=w736, "error in"=w735) -> ("task out"=w791:refnum<k21>, "error out"=w790:errorcluster)  [unwired: 10 in, 1 out]
            n217 = call-poly <vilib>:"DAQmx Read.vi"("task/channels in"=w774, "error in"=w734) -> ("task out"=w773:refnum<k21>, "data"=w733:u32, "error out"=w775:errorcluster)  [unwired: 11 in]
            "CW" <- w733
            n218 = call-poly <vilib>:"DAQmx Read.vi"("task/channels in"=w776, "error in"=w731) -> ("task out"=w778:refnum<k21>, "data"=w732:u32, "error out"=w777:errorcluster)  [unwired: 11 in]
            "CCW" <- w732
            n219 = case shown="True" "LL (M - A)" {
              tunnel: [w800 w810] -> w757
              tunnel: [w801 w809] -> w756
              tunnel: w755 -> [w803 w808]
              tunnel: [w799 w807] -> w754
              tunnel: w753 -> [_ w806]
              tunnel: "Lid Lock Feedback" -> [w802 _]
              tunnel: w723 -> [w799 w805]
              tunnel: w720 -> [w798 w804]
              frame False {
                n220 = call-poly <vilib>:"DAQmx Write.vi"("task/channels in"=w803, "data"=w802, "error in"=w798) -> ("task out"=w801:refnum<k21>, "error out"=w800:errorcluster)  [unwired: 10 in, 1 out]
              }
              frame True {
                # "Automatic Lid Lock feedback"
                n221 = case shown="True" w806 {
                  tunnel: w808 -> [w816 w819]
                  tunnel: [w815 w818] -> w810
                  tunnel: [w814 w819] -> w809
                  tunnel: [w813 w817] -> w807
                  tunnel: w805 -> [w812 w817]
                  tunnel: w804 -> [w811 w818]
                  frame False {
                    n222 = Not(x=w812) -> (.not. x?=w813:bool)
                    n223 = call-poly <vilib>:"DAQmx Write.vi"("task/channels in"=w816, "data"=w813, "error in"=w811) -> ("task out"=w814:refnum<k21>, "error out"=w815:errorcluster)  [unwired: 10 in, 1 out]
                  }
                  frame True {
                  }
                }
              }
            }
            n224 = Index Array(array=w796) -> (element #1=w785:bool, element #2=w779:bool, element #3=w784:bool, element #4=w783:bool, element #5=w782:bool, element #6=w781:bool, element #7=w780:bool)  [unwired: 7 in]
            n225 = call "Counts to Triac Direction.vi"("CCW ctr"=w732, "CW ctr"=w733) -> ("CW"=w771:bool, "CCW"=w772:bool)  [unwired: 8 in]
            n226 = case shown="False" w746 {
              tunnel: w749 -> [w842 w844]
              tunnel: w748 -> [w841 w843]
              tunnel: [w840 w844] -> w787
              tunnel: [w839 w843] -> w786
              tunnel: w729 -> [w838 _]
              tunnel: w728 -> [w837 _]
              frame False {
                n227 = property class="DAQmx Channel"(reference=w842, error in=w841, "CO.Pulse.Freq"=w838, "CO.Pulse.DutyCyc"=w837) -> (reference out=w840:refnum<k21>, error out=w839:errorcluster)
              }
              frame True {
              }
            }
            n228 = Select(t=DAQ_States_Brass."Run" ("States"), s=w719, f=DAQ_States_Brass."Shutdown" ("States")) -> (s? t:f=w767:T20)
          }
          frame "Shutdown" {
            w885 = 0.0
            w882 = FALSE ("element")
            # "Hall Sensor"
            # "Motor TRIAC CCW"
            # "Motor TRIAC CW"
            # "Relay Controls"
            # "TRIAC Outputs"
            # "AO for ADC"
            n229 = local read "AC Power"() -> (w870:bool)
            n230 = Build Array(w870, w882, w882) -> (w897:bool[])
            n231 = Build Array(w885, w885, w885) -> (w884:dbl[])
            n232 = call-poly <vilib>:"DAQmx Write.vi"("task/channels in"=w896, "data"=w897, "error in"=w869) -> ("task out"=w890:refnum<k21>, "error out"=w891:errorcluster)  [unwired: 10 in, 1 out]
            n233 = call-poly <vilib>:"DAQmx Write.vi"("task/channels in"=w877, "data"=FALSE, "error in"=w846) -> ("task out"=w876:refnum<k21>, "error out"=w875:errorcluster)  [unwired: 10 in, 1 out]
            n234 = call-poly <vilib>:"DAQmx Write.vi"("task/channels in"=w893, "data"=w884, "error in"=w854) -> ("task out"=w895:refnum<k21>, "error out"=w894:errorcluster)  [unwired: 10 in, 1 out]
            n235 = call "Time Delay4"("error in (no error)"=w891, "Delay Time (s)"=2.0) -> ("error out"=w889:errorcluster)  [unwired: 9 in]
            n236 = call <vilib>:"DAQmx Clear Task.vi"("task in"=w881, "error in"=w847) -> ("error out"=w880:errorcluster)  [unwired: 13 in]
            n237 = call <vilib>:"DAQmx Clear Task.vi"("task in"=w845, "error in"=w871) -> ("error out"=w902:errorcluster)  [unwired: 13 in]
            n238 = call <vilib>:"DAQmx Clear Task.vi"("task in"=w890, "error in"=w889) -> ("error out"=w868:errorcluster)  [unwired: 13 in]
            n239 = call <vilib>:"DAQmx Clear Task.vi"("task in"=w895, "error in"=w894) -> ("error out"=w861:errorcluster)  [unwired: 13 in]
            n240 = call <vilib>:"DAQmx Clear Task.vi"("task in"=w887, "error in"=w853) -> ("error out"=w886:errorcluster)  [unwired: 13 in]
            n241 = call <vilib>:"DAQmx Clear Task.vi"("task in"=w899, "error in"=w852) -> ("error out"=w888:errorcluster)  [unwired: 13 in]
            n242 = call <vilib>:"DAQmx Clear Task.vi"("task in"=w900, "error in"=w851) -> ("error out"=w850:errorcluster)  [unwired: 13 in]
            n243 = call <vilib>:"DAQmx Clear Task.vi"("task in"=w876, "error in"=w875) -> ("error out"=w879:errorcluster)  [unwired: 13 in]
            n244 = property on="Motor Current" class="Slide (strict)"(error in=w861, "Value"=2.5 ("Motor Current")) -> (error out=w859:errorcluster)  [unwired: 1 in, 1 out]
            n245 = property on="Turn On DAQ" class="Bool (strict)"(error in=w868, "Value"=FALSE ("Turn On DAQ")) -> (error out=w866:errorcluster)  [unwired: 1 in, 1 out]
            n246 = property on="Basket RPM" class="DigNum (strict)"(error in=w850, "Value"=1.0 ("Basket RPM")) -> (error out=w849:errorcluster)  [unwired: 1 in, 1 out]
            n247 = property on="Temperature" class="Slide (strict)"(error in=w859, "Value"=2.5 ("Temperature")) -> (error out=w857:errorcluster)  [unwired: 1 in, 1 out]
            n248 = property on="Mode Shift FB" class="Bool (strict)"(error in=w866, "Value"=FALSE ("Mode Shift FB")) -> (error out=w864:errorcluster)  [unwired: 1 in, 1 out]
            n249 = property on="Lid Status" class="Bool (strict)"(error in=w864, "Value"=FALSE ("Lid Status")) -> (error out=w863:errorcluster)  [unwired: 1 in, 1 out]
            n250 = property on="Pressure" class="Slide (strict)"(error in=w857, "Value"=0.0 ("Pressure")) -> (error out=w856:errorcluster)  [unwired: 1 in, 1 out]
          }
          frame "Exit" {
            w920 = FALSE ("element")
            w938 = 0.0
            n251 = local read "AC Power"() -> (w921:bool)
            n252 = Build Array(w921, w920, w920) -> (w917:bool[])
            n253 = call-poly <vilib>:"DAQmx Write.vi"("task/channels in"=w913, "data"=w917, "error in"=w916) -> ("task out"=w914:refnum<k21>, "error out"=w919:errorcluster)  [unwired: 10 in, 1 out]
            n254 = Build Array(w938, w938, w938) -> (w941:dbl[])
            n255 = call-poly <vilib>:"DAQmx Write.vi"("task/channels in"=w925, "data"=FALSE, "error in"=w924) -> ("task out"=w923:refnum<k21>, "error out"=w922:errorcluster)  [unwired: 10 in, 1 out]
            n256 = call-poly <vilib>:"DAQmx Write.vi"("task/channels in"=w940, "data"=w941, "error in"=w939) -> ("task out"=w937:refnum<k21>, "error out"=w936:errorcluster)  [unwired: 10 in, 1 out]
            n257 = call "Time Delay"("error in (no error)"=w919, "Delay Time (s)"=2.0) -> ("error out"=w915:errorcluster)  [unwired: 9 in]
            n258 = case shown="True" w949 {
              tunnel: w914 -> [_ w1001]
              tunnel: w969 -> [_ w1000]
              tunnel: [w973 w999] -> w928
              tunnel: [w974 w998] -> w968
              tunnel: [w970 w997] -> w908
              tunnel: [w976 w996] -> w911
              tunnel: [w977 w995] -> w967
              tunnel: w963 -> [_ w994]
              tunnel: w962 -> [_ w993]
              tunnel: [w975 w992] -> w961
              tunnel: w959 -> [_ w991]
              tunnel: [w972 w990] -> w958
              tunnel: w923 -> [_ w989]
              tunnel: [w971 w988] -> w906
              tunnel: w954 -> [w977 w987]
              tunnel: w915 -> [w976 w986]
              tunnel: w953 -> [w975 w985]
              tunnel: w952 -> [w974 w984]
              tunnel: w951 -> [w973 w983]
              tunnel: w950 -> [w972 w982]
              tunnel: w922 -> [w971 w981]
              tunnel: w948 -> [_ w980]
              tunnel: w937 -> [_ w979]
              tunnel: w936 -> [w970 w978]
              frame False {
              }
              frame True {
                # "Hall Sensor"
                # "Motor TRIAC CCW"
                # "Motor TRIAC CW"
                # "Relay Controls"
                # "TRIAC Outputs"
                # "AO for ADC"
                n259 = call <vilib>:"DAQmx Clear Task.vi"("task in"=w991, "error in"=w982) -> ("error out"=w990:errorcluster)  [unwired: 13 in]
                n260 = call <vilib>:"DAQmx Clear Task.vi"("task in"=w989, "error in"=w981) -> ("error out"=w988:errorcluster)  [unwired: 13 in]
                n261 = call <vilib>:"DAQmx Clear Task.vi"("task in"=w980, "error in"=w987) -> ("error out"=w995:errorcluster)  [unwired: 13 in]
                n262 = call <vilib>:"DAQmx Clear Task.vi"("task in"=w1001, "error in"=w986) -> ("error out"=w996:errorcluster)  [unwired: 13 in]
                n263 = call <vilib>:"DAQmx Clear Task.vi"("task in"=w979, "error in"=w978) -> ("error out"=w997:errorcluster)  [unwired: 13 in]
                n264 = call <vilib>:"DAQmx Clear Task.vi"("task in"=w993, "error in"=w985) -> ("error out"=w992:errorcluster)  [unwired: 13 in]
                n265 = call <vilib>:"DAQmx Clear Task.vi"("task in"=w994, "error in"=w984) -> ("error out"=w998:errorcluster)  [unwired: 13 in]
                n266 = call <vilib>:"DAQmx Clear Task.vi"("task in"=w1000, "error in"=w983) -> ("error out"=w999:errorcluster)  [unwired: 13 in]
              }
            }
            n267 = call <vilib>:"Clear Errors.vi"("error in (no error)"=w908, "specific error code to clear (0: all)"=-200088) -> ("error out"=w907:errorcluster)  [unwired: 4 in, 1 out]
            n268 = call <vilib>:"Clear Errors.vi"("error in (no error)"=w911, "specific error code to clear (0: all)"=-200088) -> ("error out"=w910:errorcluster)  [unwired: 4 in, 1 out]
            n269 = call <vilib>:"Clear Errors.vi"("error in (no error)"=w906, "specific error code to clear (0: all)"=-200088) -> ("error out"=w905:errorcluster)  [unwired: 4 in, 1 out]
            n270 = property on="Turn On DAQ" class="Bool (strict)"(error in=w910, "Value"=FALSE ("Turn On DAQ")) -> (error out=w946:errorcluster)  [unwired: 1 in, 1 out]
            n271 = property on="Motor Current" class="Slide (strict)"(error in=w907, "Value"=2.5 ("Motor Current")) -> (error out=w934:errorcluster)  [unwired: 1 in, 1 out]
            n272 = property on="Basket RPM" class="DigNum (strict)"(error in=w928, "Value"=1.0 ("Basket RPM")) -> (error out=w927:errorcluster)  [unwired: 1 in, 1 out]
            n273 = property on="Mode Shift FB" class="Bool (strict)"(error in=w946, "Value"=FALSE ("Mode Shift FB")) -> (error out=w944:errorcluster)  [unwired: 1 in, 1 out]
            n274 = property on="Temperature" class="Slide (strict)"(error in=w934, "Value"=2.5 ("Temperature")) -> (error out=w932:errorcluster)  [unwired: 1 in, 1 out]
            n275 = property on="Lid Status" class="Bool (strict)"(error in=w944, "Value"=FALSE ("Lid Status")) -> (error out=w942:errorcluster)  [unwired: 1 in, 1 out]
            n276 = property on="Pressure" class="Slide (strict)"(error in=w932, "Value"=0.0 ("Pressure")) -> (error out=w930:errorcluster)  [unwired: 1 in, 1 out]
          }
        }
        "DAQ Status" <- w463
        "DAQ On?" <- w461
        "Triac CW" <- w458
        "Traic CCW" <- w457
        "Cold Valve" <- w433
        "Recirc Pump" <- w434
        "Mode Shift" <- w420
        "Drain Pump" <- w435
        "Fabric SoftValve" <- w430
        "Spray/Rinse Valve" <- w431
        "Hot Valve" <- w432
        n277 = case shown="True" "MS (M - A)" {
          tunnel: w425 -> [w487 w498]
          tunnel: [w487 w497] -> w421
          tunnel: w420 -> [_ w488]
          frame False {
          }
          frame True {
            n278 = Equal?(x=w488, y=TRUE) -> (x = y?=w495:bool)
            n279 = case shown="True" w495 {
              tunnel: w498 -> [w503 w505]
              tunnel: [w503 w504] -> w490
              frame False {
              }
              frame True {
                n280 = Increment(x=w505) -> (x+1=w504:dbl)
              }
            }
            n281 = In Range and Coerce(upper limit=24.0, x=w490, lower limit=15.0) -> (In Range?=w492:bool)  [unwired: 1 out]
            n282 = case shown="True" w492 {
              frame False {
                n283 = property on="Mode Shift FB" class="Bool (strict)"("Value"=FALSE ("Mode Shift FB")) -> ()  [unwired: 2 in, 2 out]
              }
              frame True {
                n284 = property on="Mode Shift FB" class="Bool (strict)"("Value"=TRUE ("Mode Shift FB")) -> ()  [unwired: 2 in, 2 out]
              }
            }
            n285 = Greater Or Equal?(x=w490, y=24.0) -> (x >= y?=w489:bool)
            n286 = case shown="True" w489 {
              tunnel: w490 -> [w499 _]
              tunnel: [w499 0.0] -> w497
              frame False {
              }
              frame True {
              }
            }
          }
        }
        n287 = case shown="False" w428 {
          tunnel: w426 -> [w507 _]
          tunnel: [w506 0.0] -> w422
          frame False {
            n288 = Increment(x=w507) -> (x+1=w506:dbl)
          }
          frame True {
          }
        }
        n289 = Merge Errors(w472, w471, w470, w469, w468, w467, w466, w465, w464) -> (w473:errorcluster)
        n290 = call "Error_Control_Brass.vi"("Error In"=w473) -> ("Error Out"=w485:errorcluster)  [unwired: 14 in]
      }
      n291 = while "Periodic ERD Query Loop" {
        shift-right: [w187] -> w49
        shift-left: w76 -> [w189]
        tunnel: w66 -> [w190]
        shift-right: [w184] -> _
        shift-left: _ -> [w183]
        shift-right: [w178] -> _
        shift-left: w68 -> [w180]
        shift-right: [w173] -> _
        shift-left: _ -> [w172]
        tunnel: w64 -> [w171]
        tunnel: [w170] -> w47
        shift-right: [w169] -> _
        shift-left: _ -> [w168]
        tunnel: w60 -> [w167]
        i -> [w166]
        stop <- w186 stop-if-true
        # "ERD Loop"
        n292 = Dequeue Element(queue=w190, timeout in ms (-1)=0, error in (no error)=w189) -> (element=w175:T21, timed out?=w181:bool, error out=w188:errorcluster)  [unwired: 1 out]
        n293 = Unbundle By Name(w175) -> ("State"=w165:T22)
        n294 = Select(t=w180, s=w181, f=w165) -> (s? t:f=w179:T22)
        n295 = call "FGV_GEA2_Ref.vi"("Action"=enum16{"Set Ref", "Get Ref"}."Get Ref", "Error In"=w188) -> ("GEA2 Reference Out"=w174:refnum<k24>, "Error Out"=w177:errorcluster)  [unwired: 12 in]
        n296 = case shown="\"Read ERDs\"" w179 {
          tunnel: w177 -> [w200 w208 w221 w235 w254 w290 w337 w365 w373]
          tunnel: [w192 w204 w214 w235 w252 w289 w334 w365 w373] -> w185
          tunnel: [_ _ _ _ _ _ _ _ TRUE] -> w186
          tunnel: [w199 w206 w212 w238 w258 w283 w344 w366 w371] -> w184
          tunnel: w183 -> [w199 w206 w233 w238 w258 w283 w344 w366 w371]
          tunnel: T5 {"Source"=229, "Destination"=53} ("GEA Inputs") -> [_ _ w210 _ _ w287 _ _ _]
          tunnel: [ERD_Loop_States_Brass."Build ERD Read List" ("State") ERD_Loop_States_Brass."Read ERDs" ("State") ERD_Loop_States_Brass."Update UI" ("State") ERD_Loop_States_Brass."Update Graphs" ("State") ERD_Loop_States_Brass."Read Faults" ("State") ERD_Loop_States_Brass."Log Data" ("State") ERD_Loop_States_Brass."Read ERDs" ("State") ERD_Loop_States_Brass."Pause" ("State") ERD_Loop_States_Brass."Shutdown" ("State")] -> w178
          tunnel: w174 -> [_ _ w222 _ w247 w288 _ _ _]
          tunnel: [w197 w207 w211 w240 w256 w284 w343 w363 w369] -> w173
          tunnel: w172 -> [w197 _ w211 w240 w256 w284 w343 w363 w369]
          tunnel: w171 -> [w196 w203 w219 w236 w255 w282 w342 w362 w368]
          tunnel: [w196 w203 w219 w236 w255 w282 w341 w362 w368] -> w170
          tunnel: [w195 w202 w213 w237 w246 w285 w320 w361 w367] -> w169
          tunnel: w168 -> [w195 w202 _ w237 w244 w286 w320 w361 w367]
          tunnel: w167 -> [_ _ _ _ w248 _ _ _ _]
          tunnel: w166 -> [_ _ _ _ _ _ _ _ _]
          frame "Init", Default {
            # "Set Write Header\nFGV to True"
            n297 = call "Write_Header_FGV.vi"("Write Header ? In"=TRUE, "Action"=enum16{"Get", "Set"}."Set", "Error In"=w200) -> ("Error Out"=w192:errorcluster)  [unwired: 11 in, 1 out]
          }
          frame "Build ERD Read List" {
            n298 = call "ERD_Read_List_Builder.vi"("Array"="ERD Read List", "Error In"=w208) -> ("Read ERD List"=w207:T6[], "Error Out"=w204:errorcluster)  [unwired: 16 in]
          }
          frame "Read ERDs" {
            n299 = call "Convert Read ERD List to Message.vi"("GEA Inputs"=w210, "Read ERD List"=w211, "Error In"=w221) -> ("GEA Message"=w230:T3, "Error Out"=w231:errorcluster)  [unwired: 11 in]
            n300 = call "GEA2MessageFormatter.vi"("Prefix(Send/Recv)"="SEND", "GEA2 Data In"=w230, "Error In"=w231) -> ("Output String"=w229:string, "Error Out"=w228:errorcluster)  [unwired: 11 in]
            n301 = call "GExplorer_Queue_GEA2.vi"("Output String"=w229, "error in (no error)"=w228) -> ("error out"=w226:errorcluster)  [unwired: 13 in]
            n302 = Tick Count (ms)() -> (millisecond timer value=w212:u32)
            n303 = Subtract(x=w212, y=w233) -> (x-y=→"Log Rate (ms)":u32)
            n304 = call "GEA2 Read ERD Multiple Messages.vi"("GEA2 Reference In"=w222, "Retry Count"=1, "Read Timeout (ms)"=u32 250, "GEA Inputs"=w210, "Read ERD List"=w211, "Error In"=w226, "#ERDs per message"=5, "Verify ERD Response?"=FALSE) -> ("ERD Data Out"=w209:T30[], "Error Out"=w218:errorcluster)  [unwired: 4 in, 2 out]
            n305 = call "Write_Header_FGV.vi"("Action"=enum16{"Get", "Set"}."Get", "Error In"=w218) -> ("Write Header ? Out"=w215:bool, "Error Out"=w217:errorcluster)  [unwired: 12 in]
            n306 = call "Convert_ERDs_Brass.vi"("New Header?"=w215, "Array"=w209, "Error In"=w217) -> ("All_ERD_Data_Bundled_Brass"=w213:T31, "Error Out"=w214:errorcluster)  [unwired: 11 in]
          }
          frame "Update UI" {
            n307 = Unbundle By Name(w237) -> ("Version"=→"Version":T4, "ERD_Always Show"=→"ERD_Always Show":T1)
          }
          frame "Update Graphs" {
            n308 = case shown="False" "ERD Graphing ON" {
              tunnel: w254 -> [w272 w279]
              tunnel: [w272 w278] -> w253
              tunnel: "ERD Graph Cntrl" -> [_ w277]
              tunnel: [_ w276] -> w249
              tunnel: w247 -> [_ w275]
              tunnel: w244 -> [w271 w274]
              tunnel: [w271 w273] -> w243
              frame False {
              }
              frame True {
                n309 = call "Graph ERD Read List_Brass.vi"("GEA2 Reference In"=w275, "All_Bundled_Data_Brass"=w274, "ERD Graph Cntrl"=w277, "Error In"=w279) -> ("ERD Graph  Ind"=w276:T9, "All_Bundled_Data_Brass 2"=w273:T31, "Error Out"=w278:errorcluster)  [unwired: 8 in, 1 out]
              }
            }
            n310 = case shown="True" "Graphing ON" {
              tunnel: w253 -> [w259 w270]
              tunnel: [w259 w269] -> w252
              tunnel: w249 -> [_ w267]
              tunnel: w248 -> [_ w262]
              tunnel: w243 -> [w260 w261]
              tunnel: [w260 w261] -> w246
              frame False {
              }
              frame True {
                n311 = call "Update Graphs_Brass.vi"("Select Graph"="Select Graph", "appended array"=w262, "ERD Graph  Ind 2"=w267, "All_Bundled_Data_Brass"=w261, "Error In"=w270) -> ("All Loads"=→"All Loads":u16[][], "ERD 3"=→"ERD 3":dbl, "ERD 2"=→"ERD 2":dbl, "ERD 1"=→"ERD 1":dbl, "Error Out"=w269:errorcluster)  [unwired: 6 in]
                "ERD Graph  Ind" <- w267
              }
            }
          }
          frame "Read Faults" {
            n312 = case shown="True" "Fault ON" {
              tunnel: w290 -> [w291 w300]
              tunnel: [w291 w299] -> w289
              tunnel: w288 -> [_ w298]
              tunnel: w287 -> [_ w297]
              tunnel: w286 -> [w292 w296]
              tunnel: [w292 w295] -> w285
              frame False {
              }
              frame True {
                # "0-11 Sequence\n12-22 Table"
                n313 = call "GEA2 Read ERD Multiple Messages.vi"("GEA2 Reference In"=w298, "Retry Count"=2, "Read Timeout (ms)"=u32 250 ("Read Timeout (ms) 2"), "GEA Inputs"=w297, "Read ERD List"=T6[] [{"ERD Number"=132, "Data Type"=enum."string"}, {"ERD Number"=141, "Data Type"=enum."uint32_t"}, {"ERD Number"=57374, "Data Type"=enum."string"}, {"ERD Number"=57375, "Data Type"=enum."string"}, {"ERD Number"=57376, "Data Type"=enum."string"}, {"ERD Number"=57377, "Data Type"=enum."string"}, {"ERD Number"=57378, "Data Type"=enum."string"}, {"ERD Number"=57379, "Data Type"=enum."string"}, {"ERD Number"=57380, "Data Type"=enum."string"}, {"ERD Number"=57381, "Data Type"=enum."string"}, {"ERD Number"=57382, "Data Type"=enum."string"}, {"ERD Number"=57383, "Data Type"=enum."string"}, {"ERD Number"=129, "Data Type"=enum."string"}, {"ERD Number"=57474, "Data Type"=enum."string"}, {"ERD Number"=57475, "Data Type"=enum."string"}, {"ERD Number"=57476, "Data Type"=enum."string"}, {"ERD Number"=57477, "Data Type"=enum."string"}, {"ERD Number"=57478, "Data Type"=enum."string"}, {"ERD Number"=57479, "Data Type"=enum."string"}, {"ERD Number"=57480, "Data Type"=enum."string"}, {"ERD Number"=57481, "Data Type"=enum."string"}, {"ERD Number"=57482, "Data Type"=enum."string"}, {"ERD Number"=57483, "Data Type"=enum."string"}], "Error In"=w300, "#ERDs per message"=5 ("#ERDs per message 2"), "Verify ERD Response?"=FALSE) -> ("ERD Data Out"=w305:T30[], "Error Out"=w299:errorcluster)  [unwired: 4 in, 2 out]
                n314 = Array Subset(array=w305, index=12, length=11) -> (w306:T30[])
                n315 = Array Subset(array=w305, index=0, length=12) -> (w304:T30[])
                n316 = call "Fault_Table_Read.vi"("ERD Data Out"=w306) -> ("Fault Set?"=→"Fault Status":bool, "Table Buffer Status"=→"Table Buffer Status":T13, "Fault Table String Out"=→"Fault Table Buffer":string[][], "Fault Table Array Out"=w294:T33)  [unwired: 11 in]
                n317 = call "Fault_Seq_Read.vi"("Seq ERD In"=w304) -> ("Seq Buffer Status"=→"Seq Buffer Status":T13, "String"=→"Fault Sequence Buffer":string)  [unwired: 13 in]
                n318 = Bundle By Name(cluster=w296, "Fault Table Array"=w294) -> (w295:T31)
              }
            }
          }
          frame "Log Data" {
            # "TimeStamp"
            # "Append With Fault Log Data"
            # "Write Date/Time Header"
            n319 = Unbundle By Name(w320) -> ("CSV File String Arrays.ERD Name Array"=w340:string[], "CSV File String Arrays.ERD Number Array"=w339:string[], "CSV File String Arrays.ERD Converted String Data"=w332:string[])
            n320 = call "Write_Header_FGV.vi"("Action"=enum16{"Get", "Set"}."Get", "Error In"=w337) -> ("Write Header ? Out"=w318:bool, "Error Out"=w331:errorcluster)  [unwired: 12 in]
            n321 = case shown="True" w318 {
              tunnel: w340 -> [w353 _]
              tunnel: [w355 string[] [] ("ERD Name Array")] -> w330
              tunnel: w339 -> [w354 _]
              tunnel: [w358 string[] [] ("ERD Number Array")] -> w328
              frame True {
                n322 = Insert Into Array(array=w354, index=0, new element #1="", new element #2="", new element #3="", new element #4="") -> (w358:string[])
                n323 = Insert Into Array(array=w353, index=0, new element #1="Date", new element #2="Time", new element #3="HH:MM:SS", new element #4=".SS" ("new element/subarray")) -> (w355:string[])
              }
              frame False {
              }
            }
            n324 = call "TimeStamp to String Array.vi"("String Array In"=w332) -> ("String Array Out"=w326:string[])  [unwired: 10 in]
            n325 = Unbundle By Name(w320) -> ("Fault Table Array"=w319:T33)
            n326 = call "Faults_To_String_Array.vi"("Write Header ?"=w318, "Fault Table Entry"=w319, "Error In"=w331) -> ("Fault Header String Array"=w325:string[], "Fault ERD Number String Array"=w324:string[], "Fault Data String Array"=w323:string[], "Error Out"=w321:errorcluster)  [unwired: 13 in]
            n327 = Insert Into Array(array=w330, new element=w325) -> (w329:string[])  [unwired: 1 in]
            n328 = Insert Into Array(array=w328, new element=w324) -> (w327:string[])  [unwired: 1 in]
            n329 = Insert Into Array(array=w326, new element=w323) -> (w322:string[])  [unwired: 1 in]
            n330 = call "Write _To_CSV_File.vi"("Refnum In"=w342, "String Array 1"=w329, "String Array 2"=w327, "String Array 3"=w322, "Error In"=w321) -> ("Refnum Out"=w341:refnum<file>, "Error Out"=w335:errorcluster)  [unwired: 12 in, 1 out]
            n331 = call "Write_Header_FGV.vi"("Write Header ? In"=FALSE, "Action"=enum16{"Get", "Set"}."Set", "Error In"=w335) -> ("Error Out"=w334:errorcluster)  [unwired: 11 in, 1 out]
          }
          frame "Pause" {
          }
          frame "Shutdown" {
          }
        }
        n332 = call "Error_Control_Brass.vi"("Error In"=w185) -> ("Error Out"=w187:errorcluster)  [unwired: 14 in]
      }
      n333 = while "GEA2 Receive Message Loop" {
        shift-right: [w1303] -> w126
        shift-left: w32 -> [w1304]
        shift-right: [w1300] -> _
        shift-left: w115 -> [w1305]
        stop <- w1302 stop-if-true
        # "GEA2 Receive Message Loop"
        n334 = event shown="[0] <Data>: User Event" {
          selector: w1305 -> [w1321 w1323 w1339 w1345]
          dyn-events: [w1321 w1323 w1334 w1345] -> w1300
          timeout: _ -> [_ _ _ _]
          tunnel: w1304 -> [w1320 w1325 w1342 w1347]
          tunnel: [w1308 w1325 w1327 w1347] -> w1301
          tunnel: [FALSE TRUE _ TRUE] -> w1302
          event User Event {
            n335 = event-data() -> ("Source"=w1315:u8, "Destination"=w1314:u8, "Command"=w1313:u8, "Message"=w1312:string)  [unwired: 1 in]
            n336 = Bundle By Name(cluster=T3 {"Source"=0, "Destination"=0, "Command"=0, "Message"=""} ("GEA2 Msg"), "Source"=w1315, "Destination"=w1314, "Command"=w1313, "Message"=w1312) -> (w1306:T3)
            n337 = call "GEA2 Log Filter.vi"("Filter Log"="Filter Log", "Filter Data"="Filter Data", "GEA2 Msg"=w1306, "Cmd to Filter"="Cmd", "error in (no error)"=w1320) -> ("error out"=w1309:errorcluster)  [unwired: 10 in]
            n338 = call "FGV_GEA2_Ref.vi"("Action"=enum16{"Set Ref", "Get Ref"}."Get Ref", "Error In"=w1309) -> ("GEA2 Reference Out"=w1307:refnum<k24>, "Error Out"=w1310:errorcluster)  [unwired: 12 in]
            n339 = call "ACK Subscriptions Publications.vi"("GEA2 Reference In"=w1307, "GEA2 Msg"=w1306, "error in (no error)"=w1310) -> ("error out"=w1308:errorcluster)  [unwired: 11 in, 1 out]
          }
          event User Event {
            n340 = event-data() -> ()  [unwired: 1 in, 1 out]
          }
          event "Board Index": Value Change {
            # "Stop old GEA2\nbus reference"
            # "Allow other references a chance\nto begin using new reference"
            # "Store new GEA2 bus reference"
            # "Update event registration\nand initialize new GEA2 bus"
            # "Get the previous GEA2\nbus ref, but don't stop it\nuntil we update the FGV\nwith the new GEA2 ref"
            n341 = event-data() -> ("NewVal"=w1338:u8)  [unwired: 1 in]
            n342 = property on="Board Index" class="DigNum (strict)"(error in=w1342, "DisabledEnum"=T28."Disabled and Grayed Out" ("Disabled")) -> (error out=w1343:errorcluster)  [unwired: 1 in, 1 out]
            n343 = call "FGV_GEA2_Ref.vi"("Action"=enum16{"Set Ref", "Get Ref"}."Get Ref", "Error In"=w1343) -> ("GEA2 Reference Out"=w1326:refnum<k24>, "Error Out"=w1340:errorcluster)  [unwired: 12 in]
            n344 = call "GEA2_Reregister.vi"("Board Index"=w1338, "Event Registration In"=w1339, "Error In"=w1340) -> ("GEA2 Reference Out"=w1332:refnum<k24>, "Board ID"=w1335:string, "Event Registration Out"=w1334:refnum<event-registration>, "Error Out"=w1336:errorcluster)  [unwired: 9 in]
            n345 = property on="Board Index" class="DigNum (strict)"(error in=w1336, "DisabledEnum"=T28."Enabled" ("Disabled")) -> (error out=w1333:errorcluster)  [unwired: 1 in, 1 out]
            n346 = local write "Board ID"(w1335) -> ()
            n347 = call "FGV_GEA2_Ref.vi"("GEA2 Reference In"=w1332, "Action"=enum16{"Set Ref", "Get Ref"}."Set Ref", "Error In"=w1333) -> ("Error Out"=w1329:errorcluster)  [unwired: 11 in, 1 out]
            n348 = call "Time Delay"("error in (no error)"=w1329, "Delay Time (s)"=3.0) -> ("error out"=w1328:errorcluster)  [unwired: 9 in]
            n349 = call "GEA2 Stop.vi"("GEA2 Reference In"=w1326, "Error In"=w1328) -> ("Error Out"=w1327:errorcluster)  [unwired: 13 in]
          }
          event "Stop": Value Change {
            n350 = event-data() -> ()  [unwired: 1 in, 6 out]
          }
        }
        n351 = call "Error_Control_Brass.vi"("Error In"=w1301) -> ("Error Out"=w1303:errorcluster)  [unwired: 14 in]
      }
      n352 = while "Continuous Send Loop" {
        shift-right: [w140] -> _
        shift-left: Cont_Send_States."Run" ("State") -> [w139]
        tunnel: w37 -> [w141]
        tunnel: [w134] -> _
        shift-right: [w132] -> w41
        shift-left: w32 -> [w143]
        stop <- w142 stop-if-true
        # "Continuous Send Loop"
        n353 = Dequeue Element(queue=w141, timeout in ms (-1)=0, error in (no error)=w143) -> (queue out=w135:refnum<queue>, element=w128:T17, timed out?=w136:bool, error out=w131:errorcluster)
        n354 = Select(t=w139, s=w136, f=w128) -> (s? t:f=w138:T17)
        n355 = property on="GEA2 Send" class="Clust (strict)"() -> ("Value"=w130:T3)  [unwired: 2 in, 2 out]
        n356 = case shown="\"Run\", Default" w138 {
          selector: w138 -> [w147 w162]
          tunnel: w131 -> [w149 w164]
          tunnel: [w148 w164] -> w133
          tunnel: [_ TRUE] -> w142
          tunnel: [w147 w162] -> w140
          tunnel: w135 -> [w146 w161]
          tunnel: [w146 w161] -> w134
          tunnel: w130 -> [w145 _]
          frame "Run", Default {
            n357 = case shown="True" "Start Send" {
              tunnel: w149 -> [w150 w153]
              tunnel: [w150 w157] -> w148
              tunnel: w145 -> [_ w155]
              frame False {
              }
              frame True {
                n358 = call "FGV_GEA2_Ref.vi"("Action"=enum16{"Set Ref", "Get Ref"}."Get Ref", "Error In"=w153) -> ("GEA2 Reference Out"=w151:refnum<k24>, "Error Out"=w152:errorcluster)  [unwired: 12 in]
                n359 = call "GEA2MessageFormatter.vi"("Prefix(Send/Recv)"="SEND", "GEA2 Data In"=w155, "Error In"=w152) -> ("Output String"=w156:string, "Error Out"=w160:errorcluster)  [unwired: 11 in]
                n360 = call "GExplorer_Queue_GEA2.vi"("Output String"=w156, "error in (no error)"=w160) -> ("error out"=w158:errorcluster)  [unwired: 13 in]
                n361 = call "GEA2 Send Message.vi"("GEA2 Reference In"=w151, "Input Data"=w155, "Error In"=w158) -> ("Error Out"=w157:errorcluster)  [unwired: 11 in, 1 out]
              }
            }
          }
          frame "Shutdown" {
          }
        }
        n362 = call "Error_Control_Brass.vi"("Error In"=w133) -> ("Error Out"=w132:errorcluster)  [unwired: 14 in]
        n363 = Wait (ms)(milliseconds to wait="Msg Rate (ms)") -> ()  [unwired: 1 out]
      }
      n364 = while "GEA2 Display Loop" {
        tunnel: w67 -> [w383]
        shift-right: [w380] -> _
        shift-left: _ -> [w386]
        shift-right: [w382] -> w96
        shift-left: w31 -> [w390]
        tunnel: w29 -> [w376]
        tunnel: [w374] -> w27
        stop <- w384 stop-if-true
        # "GEA2 Display Loop"
        n365 = Dequeue Element(queue=w383, error in (no error)=w390) -> (element=w389:T19, error out=w385:errorcluster)  [unwired: 1 in, 2 out]
        n366 = Unbundle By Name(w389) -> ("Data"=w387:variant, "State"=w388:enum16{"Add to Log", "Clear", "Shutdown"})
        n367 = case shown="\"Add to Log\", Default" w388 {
          tunnel: w387 -> [w401 _ _]
          tunnel: w386 -> [w404 w409 _]
          tunnel: [w403 w409 ""] -> w381
          tunnel: w385 -> [w402 w410 w414]
          tunnel: [w399 w410 w414] -> w377
          tunnel: [FALSE TRUE FALSE] -> w384
          tunnel: [w391 _ _] -> w375
          frame "Add to Log", Default {
            n368 = Variant To Data(error in=w402, type="", Variant=w401) -> (data=w393:string, error out=w399:errorcluster)
            n369 = String Subset(string=w393, offset (0)=22, length (rest)=7 ("length (rest)")) -> (substring=w394:string)
            n370 = Equal?(x="SEND E5", y=w394) -> (x = y?=w392:bool)
            n371 = case shown="True" w392 {
              tunnel: w404 -> [w407 w408]
              tunnel: [w406 w408] -> w403
              tunnel: w393 -> [w405 _]
              tunnel: [w405 _] -> w391
              frame False {
                n372 = Concatenate Strings(w405, w407) -> (w406:string)
              }
              frame True {
              }
            }
          }
          frame "Shutdown" {
          }
          frame "Clear" {
          }
        }
        "GEA2 Log" <- w381
        n373 = call "Write _To_TXT_File.vi"("refnum"=w376, "text"=w375, "error in"=w377) -> ("refnum out"=w374:refnum<file>, "error out"=w378:errorcluster)  [unwired: 10 in, 1 out]
        n374 = call "Error_Control_Brass.vi"("Error In"=w378) -> ("Error Out"=w382:errorcluster)  [unwired: 14 in]
        n375 = String Subset(string=w381, length (rest)="GEA2 Log Length") -> (substring=w380:string)  [unwired: 1 in]
      }
      n376 = Close File(refnum=w27, error in=w96) -> (error out=w28:errorcluster)  [unwired: 1 out]
      n377 = call "GEA2 Stop.vi"("GEA2 Reference In"=w124, "Error In"=w125) -> ("Error Out"=w108:errorcluster)  [unwired: 13 in]
      n378 = Close File(refnum=w47, error in=w49) -> (error out=w48:errorcluster)  [unwired: 1 out]
      n379 = Merge Errors(w48, w28, w41, w126, w108, w95) -> (w23:errorcluster)
      n380 = Obtain Queue(name (unnamed)="Continuous Send", element data type=Cont_Send_States_Brass."Run" ("State"), error in (no error)=w23) -> (queue out=w46:refnum<queue>, error out=w45:errorcluster)  [unwired: 2 in, 1 out]
      n381 = Obtain Queue(name (unnamed)="ERD Loop", element data type=T21 {"Data"=variant, "State"=enum."Read ERDs"} ("Data"), error in (no error)=w23) -> (queue out=w103:refnum<queue>, error out=w102:errorcluster)  [unwired: 2 in, 1 out]
      n382 = Obtain Queue(name (unnamed)="GEA2", element data type=T19 {"Data"=variant, "State"=enum."Add to Log"} ("Data"), error in (no error)=w23) -> (queue out=w112:refnum<queue>, error out=w111:errorcluster)  [unwired: 2 in, 1 out]
      n383 = Obtain Queue(name (unnamed)="DAQ", element data type=DAQ_States_Brass."Wait for Init" ("States"), error in (no error)=w23) -> (queue out=w98:refnum<queue>, error out=w99:errorcluster)  [unwired: 2 in, 1 out]
      n384 = Release Queue(queue=w46, error in (no error)=w45) -> (error out=w44:errorcluster)  [unwired: 1 in, 2 out]
      n385 = Release Queue(queue=w103, error in (no error)=w102) -> (error out=w91:errorcluster)  [unwired: 1 in, 2 out]
      n386 = Release Queue(queue=w112, error in (no error)=w111) -> (error out=w92:errorcluster)  [unwired: 1 in, 2 out]
      n387 = Release Queue(queue=w98, error in (no error)=w99) -> (error out=w93:errorcluster)  [unwired: 1 in, 2 out]
      n388 = Merge Errors(w44, w91, w92, w93) -> (w90:errorcluster)
      n389 = call "Error_Control_Brass.vi"("Command (Handle Errors)"=Error_Command_Brass."Report Errors", "Error In"=w90) -> ("Error Out"=w83:errorcluster)  [unwired: 13 in]
    }
    frame Error {
    }
  }
  n390 = call <vilib>:"Simple Error Handler.vi"("error in (no error)"=w2) -> ("error out"=→"Error Out":errorcluster)  [unwired: 4 in, 4 out]
